vi "Tosca.vi"() -> ()   [LabVIEW 2020]
uses:
  Typedefs/Tosca-Control Refs.ctl
  FSM Graph VIs/LV Source/FSM Editor/FSM Editor.xctl
  Typedefs/Tosca-Thread Indicator.ctl
  FSM Graph VIs/LV Source/Classes/FSM.Graph/FSM.Graph.lvclass
  Typedefs/Tosca-State.ctl
  Typedefs/Tosca-Thread Type.ctl
  Typedefs/Tosca-General Options.ctl
  Classes/Parameters/Parameters.lvclass
  Classes/Parameters/Parameters.lvclass/Parameters.ctl
  Imaging VIs/Tosca-Imaging Mode.ctl
  Typedefs/Tosca-Schedule Mode.ctl
  Digital Input VIs/Tosca-DI Queue Data.ctl
  Digital Input VIs/Tosca-Input Event.ctl
  Digital Input VIs/Tosca-Input Criterion.ctl
  epl-vi-lib/Utility VIs/Type Defs/Logic State.ctl
  Typedefs/Tosca-Accumulator.ctl
  Classes/State/State.lvclass
  Classes/Parameters/Write Description.vi
  Classes/Parameters/Write MATLAB function.vi
  Classes/Parameters/Write Link to.vi
  Classes/Parameters/Read mode.vi
  8f5c66ef-750c-404f-9db0-703c45192de8.vi
  1561aa21-152f-4a32-afd8-a8b752fbf593.vi
  Classes/Parameters/Read Connect.vi
  Classes/Parameters/Write Connect.vi
  Classes/Parameters/Read AI.vi
  Classes/Parameters/Write AI.vi
  Classes/Parameters/Read Masker.vi
  Classes/Parameters/Read Use masker.vi
  Classes/Parameters/Write Masker.vi
  Classes/Parameters/Write Use masker.vi
  Classes/Parameters/Read Pretrial.vi
  Classes/Parameters/Read DAQ.vi
  Classes/Parameters/Write Pretrial.vi
  Classes/Parameters/Read Schedule Mode.vi
  Classes/Parameters/Read Imaging.vi
  Classes/Parameters/Write Imaging.vi
  Classes/Parameters/Read MATLAB function.vi
  Classes/Parameters/Read Input Events.vi
  Classes/Parameters/Read Flags.vi
  Classes/Parameters/Read Link to.vi
  Classes/Parameters/Write Flowchart.vi
  Sub VIs/Tosca-Globals.vi
  <vilib>/Utility/config.llb/Open Config Data.vi
  <vilib>/Utility/config.llb/Get Key Names.vi
  <vilib>/Utility/config.llb/Read Key.vi
  <vilib>/Utility/config.llb/Read Key (String).vi
  epl-vi-lib/Utility VIs/Array Manipulation VIs/String Array to Comma Separated String.vi
  <vilib>/Utility/error.llb/Error Cluster From Error Code.vi
  <vilib>/Utility/config.llb/Close Config Data.vi
  epl-vi-lib/Signal Synthesis VIs/4th Generation/Classes/SignalManager/SignalManager.lvclass
  epl-vi-lib/Signal Synthesis VIs/4th Generation/Classes/Channel/Channel.lvclass
  <vilib>/Platform/browser.llb/Open URL in Default Browser (path).vi
panel:
  out "play":bool
  in  "Link to":path
  out "FSM.Graph":refnum<class "FSM.Graph.lvclass">(xcontrol)
  in  "Pause":bool
  out "startAI":bool
  out "AI":errorcluster
  in  "Scripting":bool
  in  "Connect":bool
  in  "Sched:Seq":bool
  in  "Sched:2AFC":bool
  in  "Sched:CS+/CS-":bool
  in  "MATLAB function":path caption="MATLAB analysis function"
  out "2P":errorcluster
  out "FrameRate":dbl format="2P: %.5f Hz"
  out "Thread Indicators":T1[](array[typedef])
  out "DI dummy":picture
  in  "Cancel":bool
  in  "Apply":bool
  in  "Save as":bool
  in  "Analog Input":bool
  out "DI":errorcluster
  in  "Status":enum32{"CSStatus", "Adapt"}(tab)
  out "Slide":i32(slide) caption="Block 1/70:" scale=0.0..9.0
  out "Log":string
  in  "Graphs":enum32{"CSHist", "Adapt"}(tab)
  out "Histogram":cluster{dbl[], dbl[]}[](graph)
  out "Track":cluster{dbl[], dbl[]}[](graph) caption="Track1"
  out "finished":errorcluster
  in  "Imaging":bool
  out "SC":string
  in  "Masker":bool
  in  "Session Info":T2={"Subject ID"="", "Session"=1, "Path"=path "", "Run"=0} {"Session" min=1 step=1}
  in  "Notes":string
  in  "Result":string
  out "Control Refs":T3
  in  "General Options":bool
  in  "Play":bool
  in  "Flowchart":bool
  in  "Calibration":bool
  in  "Devices":bool
  in  "Save":bool
  in  "Open":bool
  in  "Exit":bool
  in  "Description":string
  in  "Parameter file":path
  out "Run":i32
  in  "Stop":bool
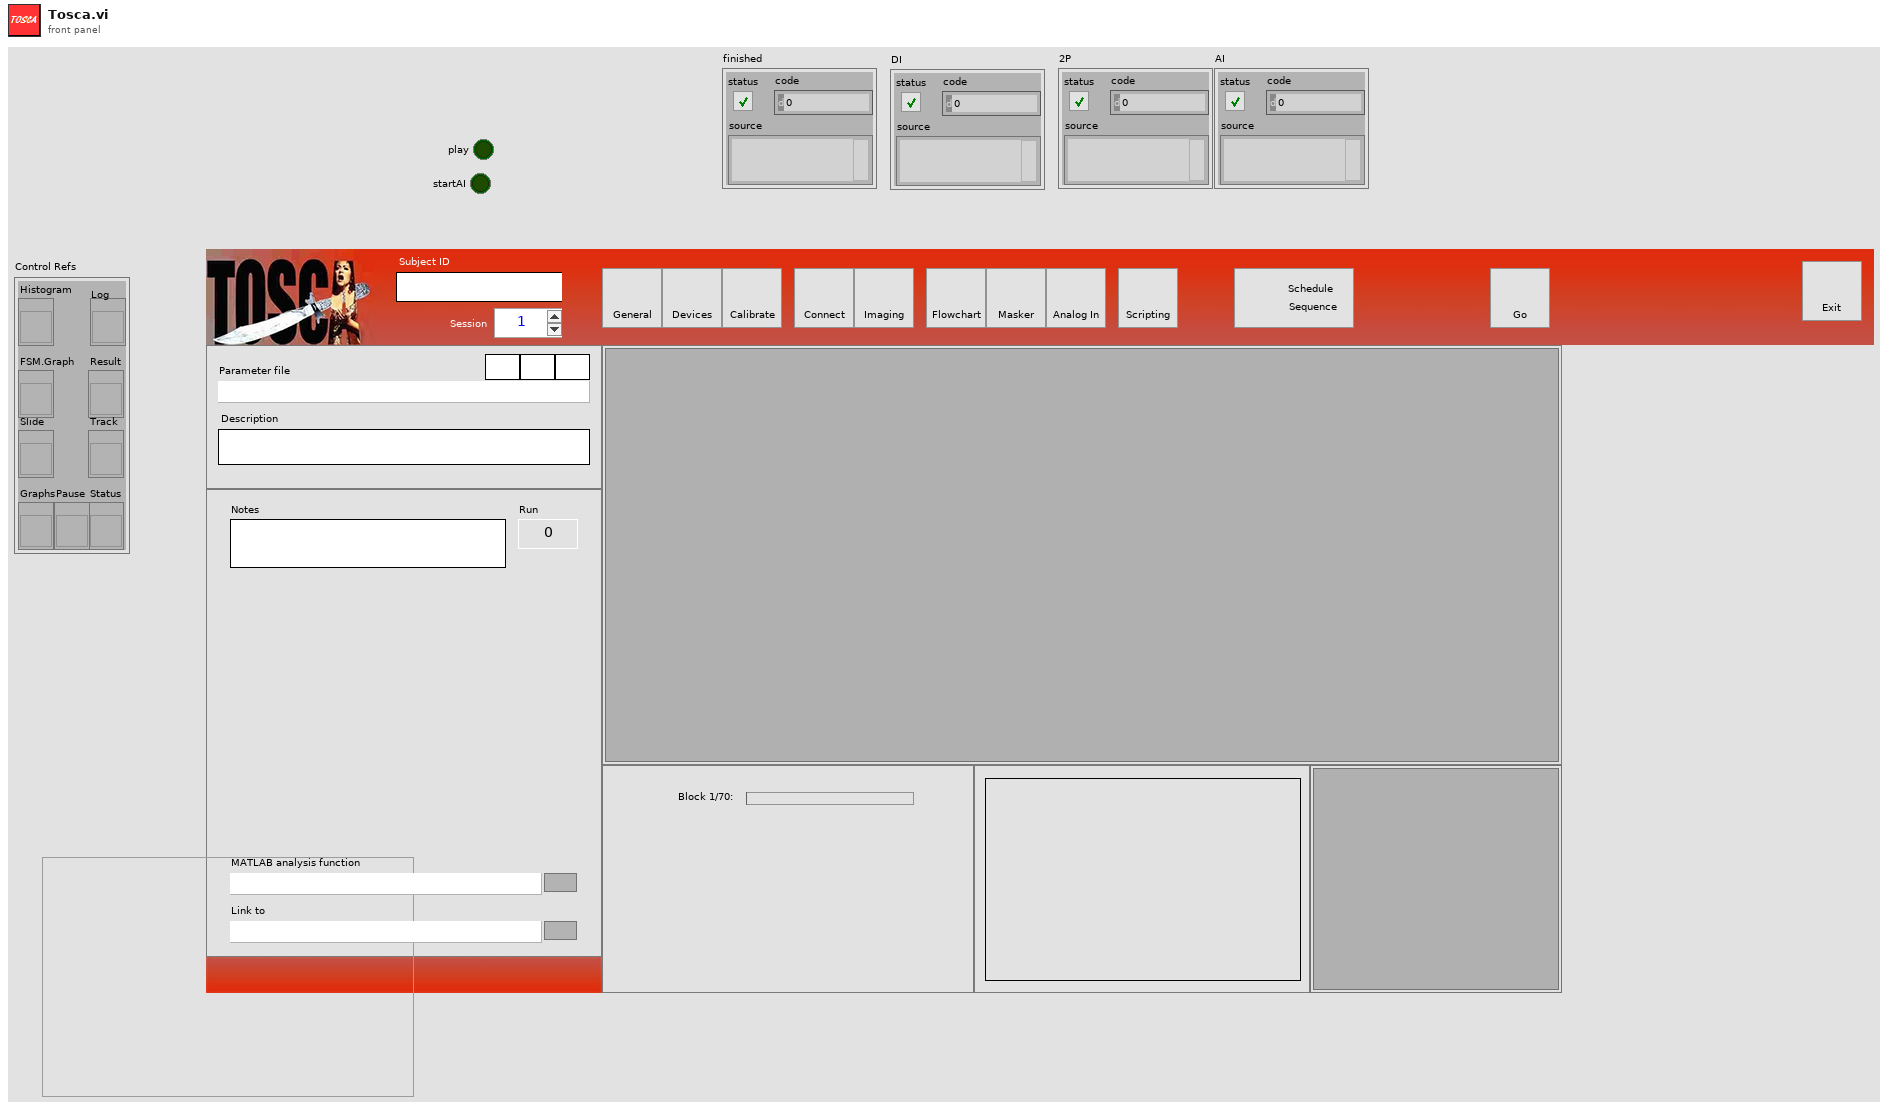
[diagram p1: front panel]
types:
  T1 = typedef "Tosca-Thread Indicator.ctl" = u16
  T2 = cluster{"Subject ID":string, "Session":i32, "Path":path, "Run":i32}
  T3 = typedef "Tosca-Control Refs.ctl" = cluster{"FSM.Graph":refnum<vi>, "Slide":refnum<vi>, "Result":refnum<vi>, "Histogram":refnum<vi>, "Graphs":refnum<vi>, "Track":refnum<vi>, "Log":refnum<vi>, "Status":refnum<vi>, "Pause":refnum<vi>}
  T4 = typedef "Tosca-State.ctl" = cluster{"Measuring":bool, "DI running":bool, "dirty":bool, "Restore":cluster{"Params":path}, "Session":cluster{"ID":string, "Num":i32, "Path":path, "Run":i32}, "active threads":T5[], "MATLAB":bool, "Config":path, "aborted":bool}
  T5 = typedef "Tosca-Thread Type.ctl" = enum16{"None", "AODO", "Masker", "ET", "Imaging", "Pupil", "AI", "DI", "Camera", "TTL out", "Loco", "Visual"}
  T6 = typedef "Tosca-IPC.ctl" = cluster{"Start":refnum<notifier>, "DI":refnum<queue>, "AO/DO":refnum<queue>, "Synapse":refnum<queue>, "Message":refnum<queue>, "Abort":refnum<notifier>, "Events":cluster{"DI":refnum<user-event>, "Threads ":refnum<user-event>}, "T/S/R":refnum<notifier>, "2P":refnum<notifier>, "MATLAB":refnum<notifier>, "Pupil":refnum<queue>, "Loco":refnum<queue>, "AI":refnum<queue>, "Tracking":refnum<queue>, "Visual":refnum<queue>, "File":refnum<notifier>}
  T7 = typedef "Tosca-2P-Notifier Data.ctl" = cluster{"Start":bool}
  T8 = typedef "Tosca-DI Queue Data.ctl" = cluster{"Action":enum16{"Stop", "Preview", "Run"}, "Input Events":T9[]}
  T9 = typedef "Tosca-Input Event.ctl" = cluster{"Name":string, "Criteria":T10[], "Operators":enum16{"AND", "OR"}[], "Accumulator":T12}
  T10 = typedef "Tosca-Input Criterion.ctl" = cluster{"DigInput":i32, "State":T11, "Time (ms)":i32, "Name":string}
  T11 = typedef "Logic State.ctl" = enum16{"Low", "High", "Rising", "Falling"}
  T12 = typedef "Tosca-Accumulator.ctl" = cluster{"active":bool, "N":i32, "T":dbl, "Imax":dbl, "latency":dbl}
  T13 = typedef "Tosca-State AODO.ctl" = cluster{"Name":string, "T (s)":dbl, "First AO":dbl[][], "frames/rep":i32, "finish?":bool, "Nrep":i32, "AO":T14, "DO":T15, "immediate":bool, "First DO":bool[][], "SigMan":refnum<class "SignalManager.lvclass">}
  T14 = typedef "Tosca-AO Runtime.ctl" = cluster{"Fs (Hz)":dbl, "pts/frame":i32, "pts/rep":i32, "ramp off":bool[], "fade out":dbl[][]}
  T15 = typedef "Tosca-DO Runtime.ctl" = cluster{"Fs (Hz)":dbl, "pts/frame":i32, "pts/rep":i32, "Rep":i32, "State":i32, "Trial":i32, "Frame":i32, "frOut":bool[], "Nchan":i32}
  T16 = typedef "Tosca-Synapse Start Data.ctl" = cluster{"Path":path, "Codes":string, "retrieve":bool}
  T17 = typedef "Tosca-SG Runtime Params.ctl" = cluster{"AO":T14, "DO":T15, "image":T18}
  T18 = typedef "Tosca-Imaging Mode.ctl" = enum16{"Off", "Widefield", "Two-photon"}
  T19 = typedef "Tosca-Session Info.ctl" = cluster{"Animal ID":string, "Session":i32, "Path":path, "Run":i32}
  T20 = typedef "Tosca-Analysis State.ctl" = cluster{"Path":path, "Attempted":i32, "Adapt":T21, "MATLAB function":path, "Results":T24[], "group order":i32[], "Connect":T25}
  T21 = typedef "Tosca-Adaptation State.ctl" = cluster{"which":i32, "nacq":i32, "Tracks":T22[]}
  T22 = typedef "Tosca-Adaptation Track State.ctl" = cluster{"Value":dbl, "Ncorrect":i32, "Nrev":i32, "Prev":dbl, "History":T23[], "Threshold":dbl, "last":i32, "type":string, "catches":dbl[][], "name":string}
  T23 = typedef "Tosca-Adaptation History Element.ctl" = cluster{"Value":dbl, "Result":string, "Log":string, "reversal":bool, "Catch":dbl}
  T24 = typedef "Parameters.lvclass/Histogram Data.ctl" = cluster{"Family":string, "Names":string[], "Colors":u32[], "N":i32[]}
  T25 = typedef "Parameters.lvclass/Connect.ctl" = cluster{"Tracking":bool, "Synapse":bool, "Pupil":bool, "Loco":bool, "Retrieve":bool, "Codes":string}
  T26 = typedef "Tosca-SCL Element.ctl" = cluster{"name":string, "vars":cluster{"state":string, "chan":string, "param":string, "value":dbl}[], "text":string, "mode":T27, "family":string, "type":T28}
  T27 = typedef "Tosca-Schedule Mode.ctl" = enum16{"Seq", "CS+/CS-", "Adapt"}
  T28 = typedef "Tosca-Event Type.ctl" = enum16{"Normal", "CS+", "CS-"}
  T29 = typedef "Tosca-Trial Result Enum.ctl" = enum16{"No trial", "Go", "No go", "Error", "Abort"}
  T30 = enum16{"big-endian, network order", "native, host order", "little-endian"}
  T31 = enum8{"Enabled", "Disabled", "Disabled and Grayed Out"}
  T32 = typedef "Tosca-General Options.ctl" = cluster{"AutoDI":bool, "Max errors":i32, "Headway (%)":dbl, "DI dt":i32}
  T33 = typedef "Tosca-Visual Display Settings.ctl" = cluster{"Use PTB":bool, "IP Address":string, "Port":i32, "rect":cluster{"left":i16, "top":i16, "width":i16, "height":i16}, "Full screen":bool, "Open at start":bool, "Monitor":i32, "Monitor size (in)":dbl, "Monitor dist (in)":dbl, "Photodiode Square":cluster{"size":i16, "location":enum16{"Bottom Left", "Top Left", "Top Right", "Bottom Right"}}, "Background":dbl}
  T34 = cluster{"FSM.Graph":refnum<vi>, "Slide":refnum<vi>, "Result":refnum<vi>, "Histogram":refnum<vi>, "Graphs":refnum<vi>, "Track":refnum<vi>, "Log":refnum<vi>, "Status":refnum<vi>, "Pause":refnum<vi>}
  T35 = cluster{"ID":string, "Num":i32, "Path":path, "Run":i32}
  T36 = typedef "Tosca-AI.ctl" = cluster{"active":bool, "Fs":dbl, "AI":string[], "DI":string[]}
  T37 = typedef "Tosca-Pretrial Spec.ctl" = cluster{"Path":path, "Args":string[]}
  T38 = typedef "Parameters.lvclass/DAQ.ctl" = cluster{"AO Fs (Hz)":dbl, "DO Fs (Hz)":dbl, "Poll Rate (Hz)":dbl, "Baseline (s)":dbl}
  T39 = typedef "Tosca-Imaging.ctl" = cluster{"mode":T18, "FrameRateHz":dbl, "use AO":bool, "destination":string}
  T40 = typedef "Tosca-Flag.ctl" = cluster{"Name":string, "Default":i32}
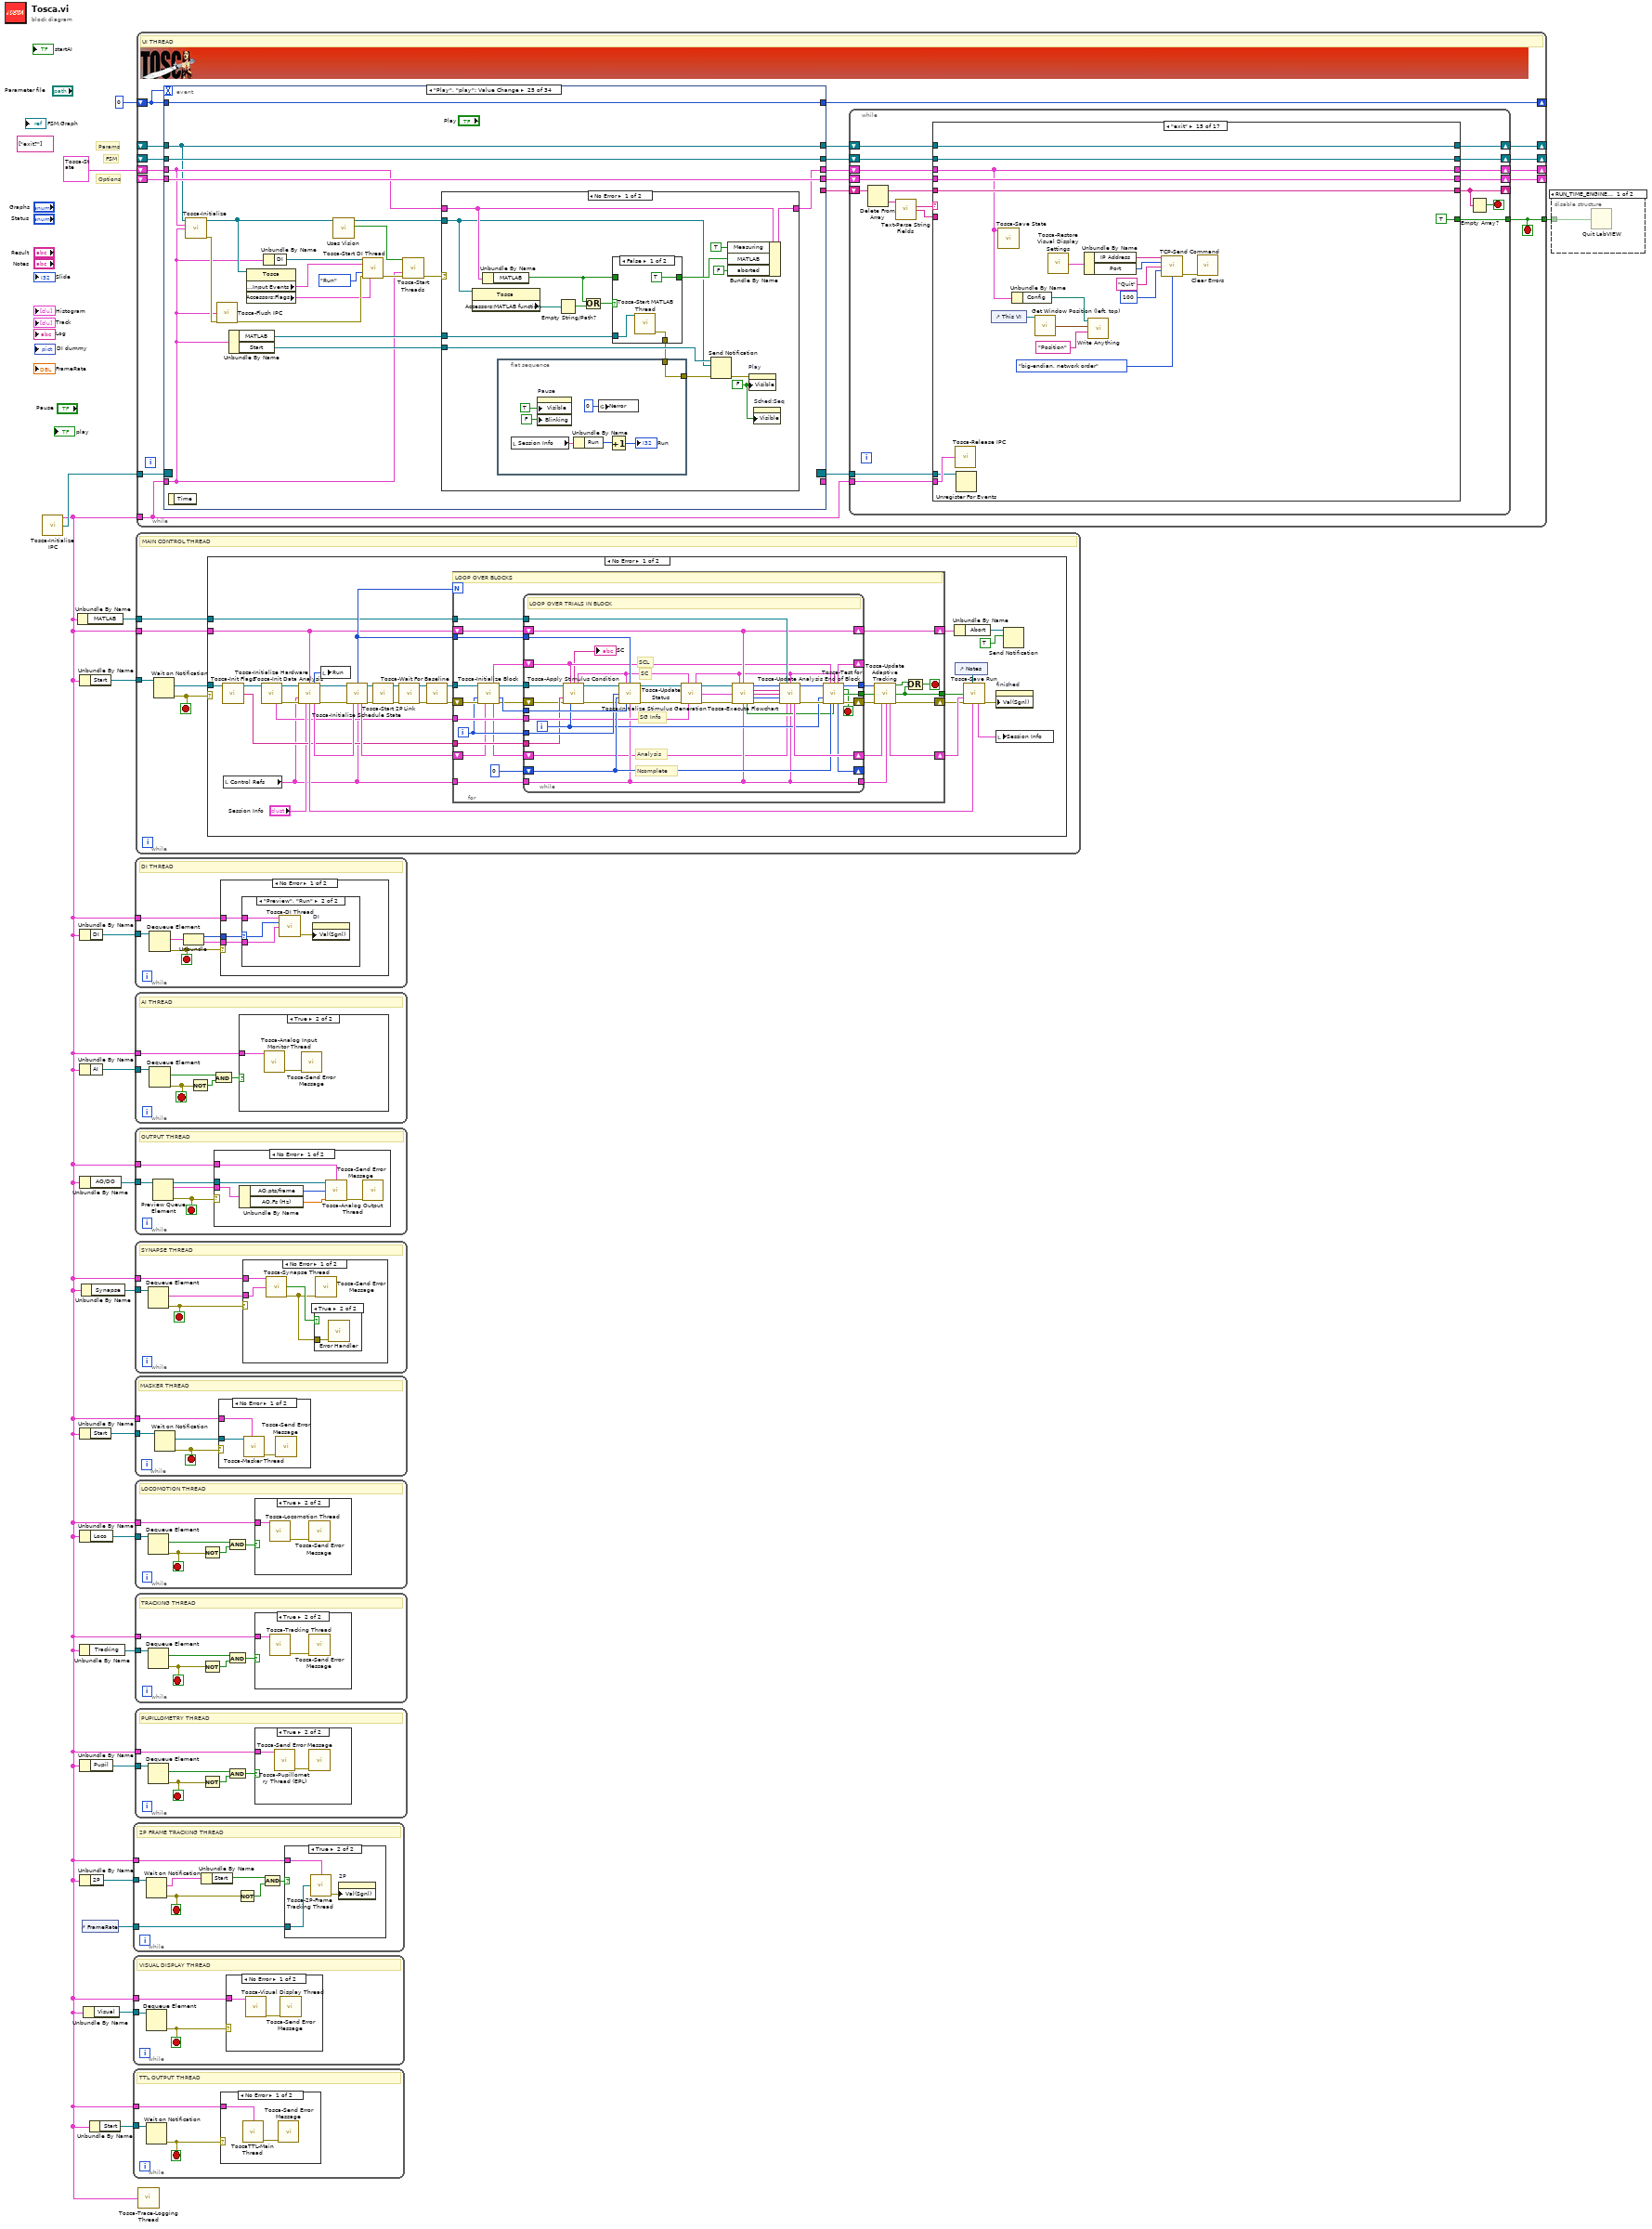
[diagram p0: block diagram]
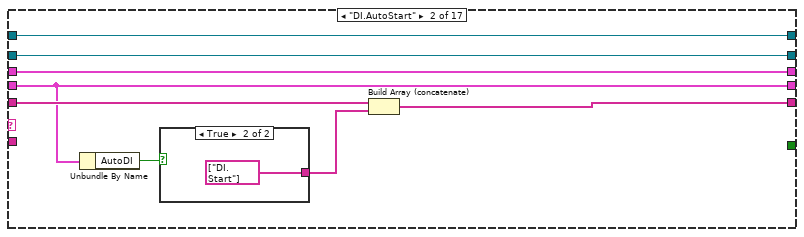
[diagram p5: hidden frame]
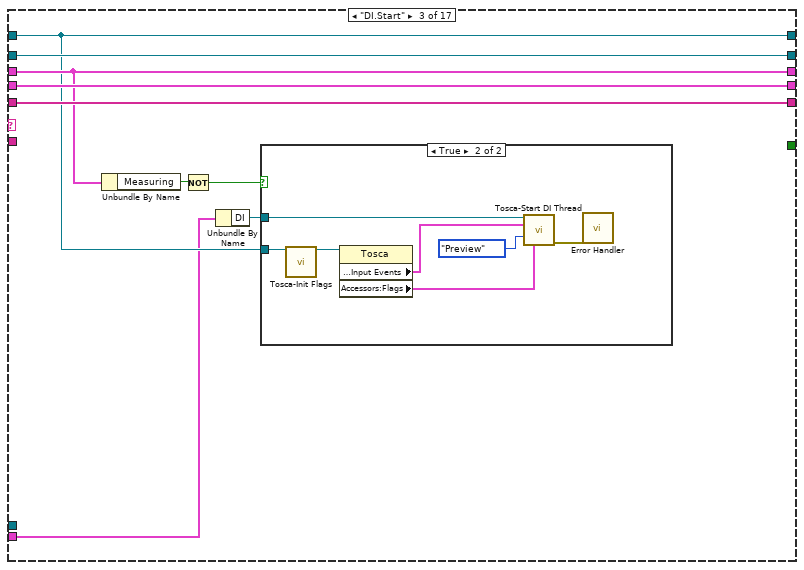
[diagram p7: hidden frame]
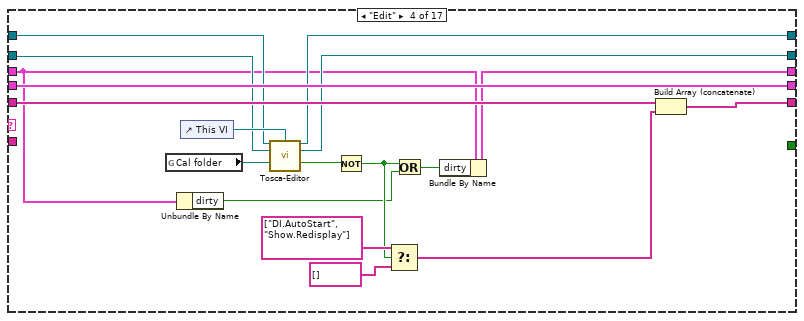
[diagram p9: hidden frame]
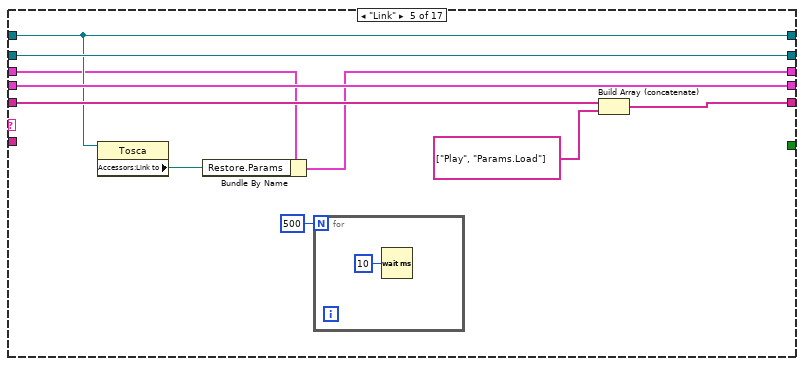
[diagram p10: hidden frame]
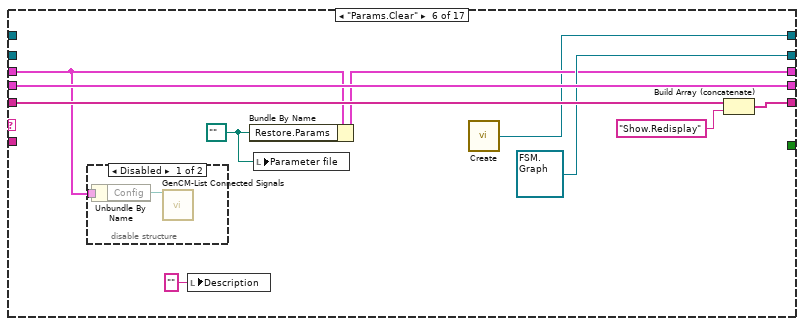
[diagram p11: hidden frame]
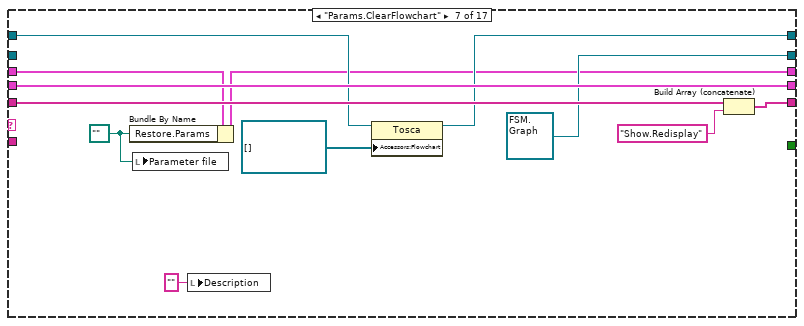
[diagram p13: hidden frame]
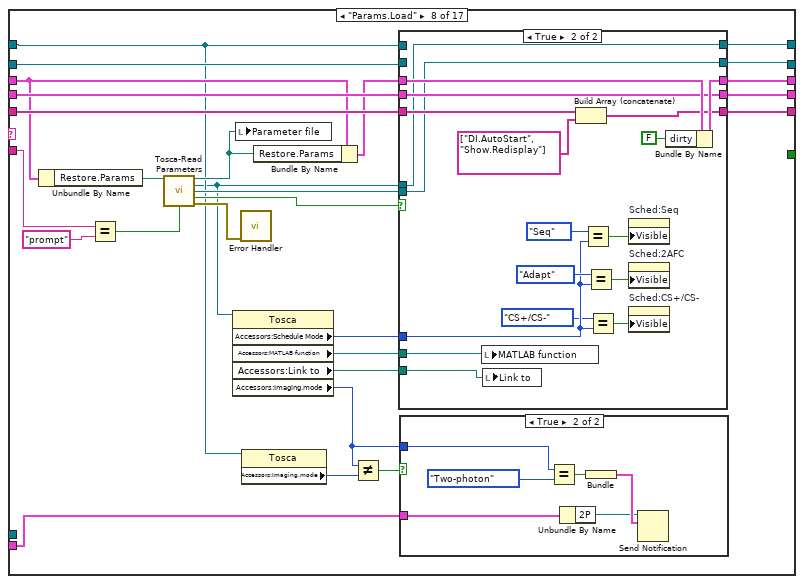
[diagram p14: hidden frame]
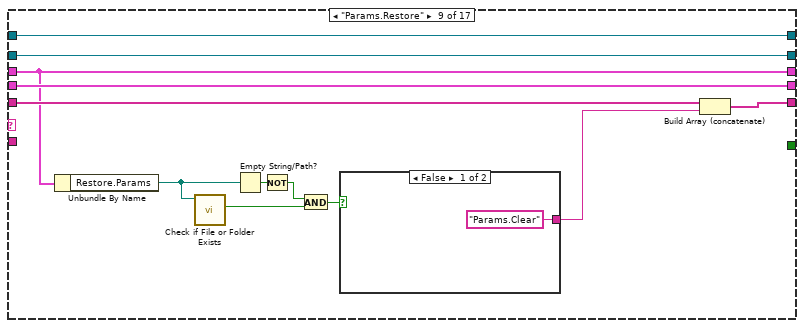
[diagram p17: hidden frame]
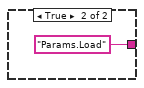
[diagram p18: hidden frame]
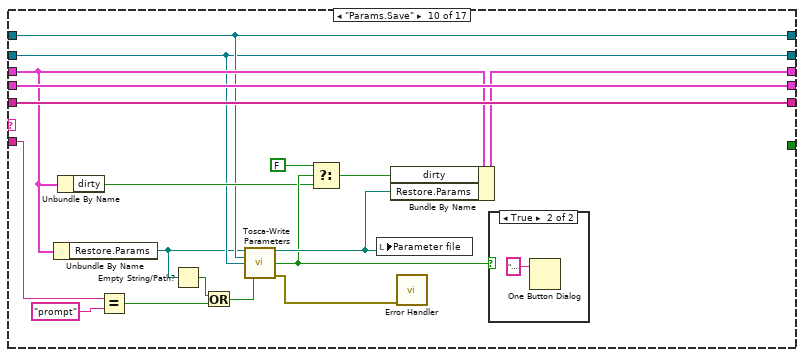
[diagram p19: hidden frame]
diagram:
  (unwired) string[] ["exit?"]
  # "FSM"
  # "Params"
  # "Options"
  n1 = call "Tosca-Initialize IPC.vi"() -> ("IPC"=w1:T6, "Event Registration Refnum"=w11:refnum<event-registration>)  [unwired: 13 in, 1 out]
  n2 = Unbundle By Name(w1) -> ("MATLAB"=w8:refnum<notifier>)
  n3 = Unbundle By Name(w1) -> ("Tracking"=w3:refnum<queue>)
  n4 = Unbundle By Name(w1) -> ("Start"=w17:refnum<notifier>)
  n5 = Unbundle By Name(w1) -> ("DI"=w14:refnum<queue>)
  n6 = Unbundle By Name(w1) -> ("AI"=w4:refnum<queue>)
  n7 = Unbundle By Name(w1) -> ("AO/DO"=w13:refnum<queue>)
  n8 = Unbundle By Name(w1) -> ("Start"=w15:refnum<notifier>)
  n9 = Unbundle By Name(w1) -> ("Loco"=w5:refnum<queue>)
  n10 = Unbundle By Name(w1) -> ("Pupil"=w6:refnum<queue>)
  n11 = Unbundle By Name(w1) -> ("2P"=w10:refnum<notifier>)
  n12 = Unbundle By Name(w1) -> ("Synapse"=w16:refnum<queue>)
  n13 = control-ref of="FrameRate"() -> (w9:refnum<vi>)
  n14 = Unbundle By Name(w1) -> ("Visual"=w2:refnum<queue>)
  n15 = Unbundle By Name(w1) -> ("Start"=w7:refnum<notifier>)
  n16 = while {
    tunnel: w10 -> [w27]
    tunnel: w1 -> [w21]
    tunnel: w9 -> [w20]
    stop <- w22 stop-if-true
    # "2P FRAME TRACKING THREAD"
    n17 = Wait on Notification(notifier=w27) -> (notification=w26:T7, error out=w22:errorcluster)  [unwired: 3 in, 2 out]
    n18 = Unbundle By Name(w26) -> ("Start"=w24:bool)
    n19 = Not(x=w22) -> (.not. x?=w23:bool)
    n20 = And(x=w24, y=w23) -> (x .and. y?=w25:bool)
    n21 = case shown="True" w25 {
      tunnel: w21 -> [_ w30]
      tunnel: w20 -> [_ w29]
      frame False {
      }
      frame True {
        n22 = call "Tosca-2P-Frame Tracking Thread.vi"("IPC"=w30, "FrameRate"=w29) -> ("error out"=w28:errorcluster)  [unwired: 13 in]
        n23 = property on="2P" class="Clust (strict)"("Val(Sgnl)"=w28) -> ()  [unwired: 2 in, 2 out]
      }
    }
  }
  n24 = while {
    tunnel: w2 -> [w33]
    tunnel: w1 -> [w32]
    stop <- w31 stop-if-true
    # "VISUAL DISPLAY THREAD"
    n25 = Dequeue Element(queue=w33) -> (error out=w31:errorcluster)  [unwired: 2 in, 3 out]
    n26 = case shown="No Error" w31 {
      tunnel: w32 -> [w34 _]
      frame No Error {
        n27 = call "Tosca-Visual Display Thread.vi"("IPC"=w34) -> ("error out"=w35:errorcluster)  [unwired: 14 in]
        n28 = call "Tosca-Send Error Message.vi"("error in (no error)"=w35) -> ()  [unwired: 15 in]
      }
      frame Error {
      }
    }
  }
  n29 = while {
    tunnel: w7 -> [w38]
    tunnel: w1 -> [w37]
    stop <- w36 stop-if-true
    # "TTL OUTPUT THREAD"
    n30 = Wait on Notification(notifier=w38) -> (error out=w36:errorcluster)  [unwired: 3 in, 3 out]
    n31 = case shown="No Error" w36 {
      tunnel: w37 -> [w40 _]
      frame No Error {
        n32 = call "ToscaTTL-Main Thread.vi"("IPC"=w40) -> ("error out"=w39:errorcluster)  [unwired: 14 in]
        n33 = call "Tosca-Send Error Message.vi"("error in (no error)"=w39) -> ()  [unwired: 15 in]
      }
      frame Error {
      }
    }
  }
  n34 = while {
    tunnel: w15 -> [w44]
    tunnel: w1 -> [w41]
    stop <- w43 stop-if-true
    # "MASKER THREAD"
    n35 = Wait on Notification(notifier=w44) -> (notification=w42:refnum<class "Parameters.lvclass">, error out=w43:errorcluster)  [unwired: 3 in, 2 out]
    n36 = case shown="No Error" w43 {
      tunnel: w42 -> [w47 _]
      tunnel: w41 -> [w45 _]
      frame No Error {
        n37 = call "Tosca-Masker Thread.vi"("IPC"=w45, "Tosca"=w47) -> ("error out"=w46:errorcluster)  [unwired: 9 in]
        n38 = call "Tosca-Send Error Message.vi"("error in (no error)"=w46) -> ()  [unwired: 15 in]
      }
      frame Error {
      }
    }
  }
  n39 = while {
    tunnel: w14 -> [w52]
    tunnel: w1 -> [w53]
    stop <- w49 stop-if-true
    # "DI THREAD"
    n40 = Dequeue Element(queue=w52) -> (element=w51:T8, error out=w49:errorcluster)  [unwired: 2 in, 2 out]
    n41 = Unbundle(w51) -> ("Action"=w48:enum16{"Stop", "Preview", "Run"}, "Input Events"=w50:T9[])
    n42 = case shown="No Error" w49 {
      tunnel: w53 -> [w56 _]
      tunnel: w50 -> [w55 _]
      tunnel: w48 -> [w54 _]
      frame No Error {
        n43 = case shown="\"Preview\", \"Run\"" w54 {
          selector: w54 -> [_ w57]
          tunnel: w56 -> [_ w60]
          tunnel: w55 -> [_ w59]
          frame "Stop", Default {
          }
          frame "Preview", "Run" {
            n44 = call "Tosca-DI Thread.vi"("IPC"=w60, "Action"=w57, "Input Events"=w59) -> ("error out"=w58:errorcluster)  [unwired: 12 in]
            n45 = property on="DI" class="Clust (strict)"("Val(Sgnl)"=w58) -> ()  [unwired: 2 in, 2 out]
          }
        }
      }
      frame Error {
      }
    }
  }
  n46 = while {
    tunnel: w4 -> [w65]
    tunnel: w1 -> [w66]
    stop <- w62 stop-if-true
    # "AI THREAD"
    n47 = Dequeue Element(queue=w65) -> (element=w63:bool, error out=w62:errorcluster)  [unwired: 2 in, 2 out]
    n48 = Not(x=w62) -> (.not. x?=w61:bool)
    n49 = And(x=w63, y=w61) -> (x .and. y?=w64:bool)
    n50 = case shown="True" w64 {
      tunnel: w66 -> [_ w68]
      frame False {
      }
      frame True {
        n51 = call "Tosca-Analog Input Monitor Thread.vi"("IPC"=w68) -> ("error out"=w67:errorcluster)  [unwired: 14 in]
        n52 = call "Tosca-Send Error Message.vi"("error in (no error)"=w67) -> ()  [unwired: 15 in]
      }
    }
  }
  n53 = while {
    tunnel: w13 -> [w73]
    tunnel: w1 -> [w71]
    stop <- w69 stop-if-true
    # "OUTPUT THREAD"
    n54 = Preview Queue Element(queue=w73) -> (queue out=w72:refnum<queue>, element=w70:T13, error out=w69:errorcluster)  [unwired: 2 in, 1 out]
    n55 = case shown="No Error" w69 {
      tunnel: w72 -> [w79 _]
      tunnel: w71 -> [w78 _]
      tunnel: w70 -> [w76 _]
      frame No Error {
        n56 = Unbundle By Name(w76) -> ("AO.pts/frame"=w75:i32, "AO.Fs (Hz)"=w74:dbl)
        n57 = call "Tosca-Analog Output Thread.vi"("Tosca Output Queue"=w79, "IPC"=w78, "pts/frame"=w75, "Fs (Hz)"=w74) -> ("error out"=w77:errorcluster)  [unwired: 11 in]
        n58 = call "Tosca-Send Error Message.vi"("error in (no error)"=w77) -> ()  [unwired: 15 in]
      }
      frame Error {
      }
    }
  }
  n59 = while {
    tunnel: w16 -> [w83]
    tunnel: w1 -> [w81]
    stop <- w82 stop-if-true
    # "SYNAPSE THREAD"
    n60 = Dequeue Element(queue=w83) -> (element=w80:T16, error out=w82:errorcluster)  [unwired: 2 in, 2 out]
    n61 = case shown="No Error" w82 {
      tunnel: w81 -> [w87 _]
      tunnel: w80 -> [w84 _]
      frame No Error {
        n62 = call "Tosca-Synapse Thread.vi"("IPC"=w87, "Data"=w84) -> ("aborted"=w86:bool, "error out"=w85:errorcluster)  [unwired: 12 in]
        n63 = case shown="True" w86 {
          tunnel: w85 -> [_ w88]
          frame False {
          }
          frame True {
            n64 = call "Error Handler.vi"("error in (no error)"=w88) -> ()  [unwired: 12 in, 3 out]
          }
        }
        n65 = call "Tosca-Send Error Message.vi"("error in (no error)"=w85) -> ()  [unwired: 15 in]
      }
      frame Error {
      }
    }
  }
  n66 = while {
    tunnel: w5 -> [w94]
    tunnel: w1 -> [w93]
    stop <- w91 stop-if-true
    # "LOCOMOTION THREAD"
    n67 = Dequeue Element(queue=w94) -> (element=w90:bool, error out=w91:errorcluster)  [unwired: 2 in, 2 out]
    n68 = Not(x=w91) -> (.not. x?=w92:bool)
    n69 = And(x=w90, y=w92) -> (x .and. y?=w89:bool)
    n70 = case shown="True" w89 {
      tunnel: w93 -> [_ w96]
      frame False {
      }
      frame True {
        n71 = call "Tosca-Locomotion Thread.vi"("IPC"=w96) -> ("error out"=w95:errorcluster)  [unwired: 14 in]
        n72 = call "Tosca-Send Error Message.vi"("error in (no error)"=w95) -> ()  [unwired: 15 in]
      }
    }
  }
  n73 = while {
    tunnel: w3 -> [w97]
    tunnel: w1 -> [w102]
    stop <- w100 stop-if-true
    # "TRACKING THREAD"
    n74 = Dequeue Element(queue=w97) -> (element=w99:bool, error out=w100:errorcluster)  [unwired: 2 in, 2 out]
    n75 = Not(x=w100) -> (.not. x?=w101:bool)
    n76 = And(x=w99, y=w101) -> (x .and. y?=w98:bool)
    n77 = case shown="True" w98 {
      tunnel: w102 -> [_ w104]
      frame False {
      }
      frame True {
        n78 = call "Tosca-Tracking Thread.vi"("IPC"=w104) -> ("error out"=w103:errorcluster)  [unwired: 14 in]
        n79 = call "Tosca-Send Error Message.vi"("error in (no error)"=w103) -> ()  [unwired: 15 in]
      }
    }
  }
  n80 = while {
    tunnel: w6 -> [w110]
    tunnel: w1 -> [w109]
    stop <- w107 stop-if-true
    # "PUPILLOMETRY THREAD"
    n81 = Dequeue Element(queue=w110) -> (element=w106:bool, error out=w107:errorcluster)  [unwired: 2 in, 2 out]
    n82 = Not(x=w107) -> (.not. x?=w108:bool)
    n83 = And(x=w106, y=w108) -> (x .and. y?=w105:bool)
    n84 = case shown="True" w105 {
      tunnel: w109 -> [_ w111]
      frame False {
      }
      frame True {
        n85 = call "Tosca-Pupillometry Thread (EPL).vi"("IPC"=w111) -> ("error out"=w112:errorcluster)  [unwired: 14 in]
        n86 = call "Tosca-Send Error Message.vi"("error in (no error)"=w112) -> ()  [unwired: 15 in]
      }
    }
  }
  n87 = while {
    tunnel: w17 -> [w117]
    tunnel: w1 -> [w114]
    tunnel: w8 -> [w113]
    stop <- w115 stop-if-true
    # "MAIN CONTROL THREAD"
    n88 = Wait on Notification(notifier=w117) -> (notification=w116:refnum<class "Parameters.lvclass">, error out=w115:errorcluster)  [unwired: 3 in, 2 out]
    n89 = case shown="No Error" w115 {
      tunnel: w116 -> [w133 _]
      tunnel: w114 -> [w119 _]
      tunnel: w113 -> [w137 _]
      frame No Error {
        n90 = call "Tosca-Init Flags.vi"("Tosca"=w133) -> ("Tosca Out"=w132:refnum<class "Parameters.lvclass">, "Names"=w135:string[])  [unwired: 13 in]
        n91 = local read "Control Refs"() -> (w118:T3)
        n92 = call "Tosca-Initialize Hardware.vi"("Tosca"=w132) -> ("Tosca out"=w130:refnum<class "Parameters.lvclass">, "SG Runtime"=w131:T17, "error out"=w124:errorcluster)  [unwired: 12 in]
        n93 = call "Tosca-Init Data Analysis.vi"("Tosca"=w130, "IPC"=w119, "Control Refs"=w118, "error in (no error)"=w124, "Session Info"="Session Info") -> ("Run"=w125:i32, "Tosca out"=w129:refnum<class "Parameters.lvclass">, "Session Info out"=w147:T19, "Analysis"=w142:T20, "error out"=w144:errorcluster)  [unwired: 6 in]
        n94 = local write "Run"(w125) -> ()
        n95 = call "Tosca-Initialize Schedule State.vi"("Tosca"=w129, "error in (no error)"=w144, "Analysis In"=w142, "Controls"=w118) -> ("Blocks"=w145:i32, "Tosca out"=w128:refnum<class "Parameters.lvclass">, "Analysis Out"=w141:T20, "error out"=w143:errorcluster)  [unwired: 8 in]
        n96 = call "Tosca-Start 2P.vi"("Tosca"=w128, "error in (no error)"=w143) -> ("Tosca out"=w127:refnum<class "Parameters.lvclass">, "error out"=w126:errorcluster)  [unwired: 12 in]
        n97 = call "Link.vi"("Tosca in"=w127, "error in (no error)"=w126) -> ("Tosca out"=w122:refnum<class "Parameters.lvclass">, "error out"=w120:errorcluster)  [unwired: 12 in]
        n98 = call "Tosca-Wait For Baseline.vi"("Parameters in"=w122, "error in (no error)"=w120) -> ("Parameters out"=w123:refnum<class "Parameters.lvclass">, "error out"=w121:errorcluster)  [unwired: 12 in]
        n99 = for {
          N: w145 -> [_]
          tunnel: w131 -> [w177]
          tunnel: w118 -> [w176]
          tunnel: w145 -> [w175]
          shift-right: [w171] -> w150
          shift-left: w141 -> [w157]
          tunnel: [w167] -> w148
          shift-right: [w169] -> w146
          shift-left: w121 -> [w178]
          shift-right: [w163] -> w140
          shift-left: w119 -> [w162]
          tunnel: w137 -> [w161]
          tunnel: w135 -> [w160]
          tunnel: w123 -> [w154]
          i -> [w159]
          stop <- w166 stop-if-true
          # "LOOP OVER BLOCKS"
          n100 = call "Tosca-Initialize Block.vi"("Tosca"=w154, "block"=w159, "error in (no error)"=w178, "Analysis in"=w157) -> ("SCL"=w152:T26[], "Tosca out"=w153:refnum<class "Parameters.lvclass">, "NumTrials"=w158:i32, "Analysis out"=w156:T20, "error out"=w155:errorcluster)  [unwired: 7 in]
          n101 = while {
            tunnel: w177 -> [w196]
            tunnel: w176 -> [w191]
            tunnel: w159 -> [w207]
            tunnel: w175 -> [w215]
            tunnel: w158 -> [w214]
            shift-right: [w211] -> w172
            shift-left: w156 -> [w190]
            tunnel: [w209] -> w170
            shift-right: [w208] -> _
            shift-left: w152 -> [w188]
            shift-right: [w204] -> _
            shift-left: 0 -> [w203]
            shift-right: [w212] -> w173
            shift-left: w155 -> [w194]
            tunnel: [w201] -> w165
            tunnel: [w191] -> w164
            shift-right: [w193] -> w163
            shift-left: w162 -> [w193]
            tunnel: w161 -> [w199]
            tunnel: w160 -> [w195]
            tunnel: w153 -> [w189]
            i -> [w200]
            stop <- w205 stop-if-true
            # "SG Info"
            # "Analysis"
            # "Ncomplete"
            # "SC"
            # "SCL"
            # "LOOP OVER TRIALS IN BLOCK"
            n102 = call "Tosca-Apply Stimulus Condition.vi"("Tosca"=w189, "SCL"=w188, "Flag names"=w195, "error in (no error)"=w194, "SCL index"=w200) -> ("text"=→"SC":string, "StimCon Element"=w180:T26, "Tosca out"=w186:refnum<class "Parameters.lvclass">, "error out"=w192:errorcluster)  [unwired: 7 in]
            n103 = call "Tosca-Update Status.vi"("StimCon"=w180, "NumBlocks"=w215, "Current Block"=w207, "This trial"=w203, "error in (no error)"=w192, "NumTrials"=w214, "Control Refs"=w191) -> ("error out"=w216:errorcluster)  [unwired: 8 in]
            n104 = call "Tosca-Initialize Stimulus Generation.vi"("Tosca"=w186, "StimCon in"=w180, "error in (no error)"=w216, "SG Runtime"=w196) -> ("StimCon out"=w179:T26, "Tosca out"=w185:refnum<class "Parameters.lvclass">, "AODO"=w184:T13[], "error out"=w181:errorcluster)  [unwired: 8 in]
            n105 = call "Tosca-Execute Flowchart.vi"("Tosca"=w185, "StimCon"=w179, "IPC"=w193, "AODO"=w184, "error in"=w181, "Control Refs"=w191) -> ("Result"=w210:T29, "History"=w202:string[], "Result string"=w198:string, "Rxn time"=w183:i32, "Abort"=w197:bool, "error out"=w182:errorcluster)  [unwired: 4 in]
            n106 = call "Tosca-Update Analysis.vi"("Result"=w210, "MATLAB"=w199, "StimCon Element"=w179, "History"=w202, "Result String"=w198, "Rxn time"=w183, "error in (no error)"=w182, "Analysis"=w190, "Control Refs"=w191) -> ("Result thru"=w206:T29, "Analysis out"=w211:T20, "error out"=w213:errorcluster)  [unwired: 4 in]
            n107 = call "Tosca-Test for End of Block.vi"("Result"=w206, "SCL in"=w188, "StimCon Element"=w179, "sclIndex"=w200, "error in (no error)"=w213, "Ncomplete"=w203, "Abort"=w197) -> ("SCL out"=w208:T26[], "Result thru"=w201:T29, "End block?"=w205:bool, "Abort?"=w209:bool, "Ncomplete out"=w204:i32, "error out"=w212:errorcluster)  [unwired: 3 in]
          }
          n108 = call "Tosca-Update Adaptive Tracking.vi"("Result"=w165, "Abort? in"=w170, "error in (no error)"=w173, "Analysis In"=w172, "Controls"=w164) -> ("Finished"=w168:bool, "Abort? out"=w167:bool, "Analysis Out"=w171:T20, "error out"=w169:errorcluster)  [unwired: 7 in]
          n109 = Or(x=w168, y=w167) -> (x .or. y?=w166:bool)
        }
        n110 = Unbundle By Name(w140) -> ("Abort"=w139:refnum<notifier>)
        n111 = control-ref of="Notes"() -> (w136:refnum<vi>)
        n112 = call "Tosca-Save Run.vi"("Notes"=w136, "Abort?"=w148, "Analysis"=w150, "error in (no error)"=w146, "Session Info"=w147) -> ("Session Info out"=w149:T19, "error out"=w151:errorcluster)  [unwired: 8 in, 1 out]
        n113 = property on="finished" class="Clust (strict)"("Val(Sgnl)"=w151) -> ()  [unwired: 2 in, 2 out]
        n114 = local write "Session Info"(w149) -> ()
        n115 = Send Notification(notification=TRUE, notifier=w139) -> ()  [unwired: 1 in, 2 out]
      }
      frame Error {
      }
    }
  }
  n116 = while {
    shift-right: [w235] -> _
    shift-left: 0 -> [w233]
    shift-right: [w220] -> _
    shift-left: _ -> [w222]
    shift-right: [w227] -> _
    shift-left: T4 {"Measuring"=FALSE, "DI running"=FALSE, "dirty"=FALSE, "Restore"={"Params"=path ""}, "Session"={"ID"="", "Num"=0, "Path"=path "", "Run"=0}, "active threads"=[], "MATLAB"=FALSE, "Config"=path "", "aborted"=FALSE} ("State") -> [w234]
    tunnel: [w225] -> w18
    tunnel: w1 -> [w223]
    shift-right: [w226] -> _
    shift-left: _ -> [w232]
    tunnel: w11 -> [w231]
    shift-right: [w218] -> _
    shift-left: _ -> [w217]
    stop <- w225 stop-if-true
    # "UI THREAD"
    n117 = event shown="[24] \"Play\", \"play\": Value Change" {
      selector: w231 -> [_ _ _ _ _ _ _ _ _ _ _ _ _ _ _ _ _ _ _ _ _ _ _ _ _ _ _ _ _ _ _ _ _ _]
      dyn-events: [_ _ _ _ _ _ _ _ _ _ _ _ _ _ _ _ _ _ _ _ _ _ _ _ _ _ _ _ _ _ _ _ _ _] -> w224
      timeout: w233 -> [_ _ _ _ _ _ _ _ _ _ _ _ _ _ _ _ _ _ _ _ _ _ _ _ _ _ _ _ _ _ _ _ _ _]
      tunnel: [-1 w602 w613 w617 w683 w687 w697 w703 w709 w715 w720 w729 w738 w747 w762 w800 w828 w859 w865 w879 w899 w918 w935 w956 w980 w1015 w1044 w1089 w1096 w1107 w1122 w1133 w1170 w1202] -> w235
      tunnel: w222 -> [_ w607 w614 w615 w682 w690 w696 w702 w708 w714 w718 w727 w736 w751 w766 w794 w830 w847 w864 w870 w894 w909 w922 w942 w966 w1018 w1031 w1088 w1095 w1106 w1121 w1132 w1152 w1201]
      tunnel: [refnum<class "Parameters.lvclass"> refnum ("Tosca") w607 w614 w615 w682 w690 w696 w702 w708 w714 w716 w725 w735 w751 w757 w795 w830 w848 w864 w866 w890 w903 w920 w936 w966 w1018 w1031 w1088 w1095 w1106 w1121 w1132 w1152 w1201] -> w221
      tunnel: w234 -> [_ w606 w611 w623 w681 w686 w695 w701 w707 w713 w724 w733 w742 w750 w765 w798 w826 w846 w862 w877 w902 w915 w933 w955 w978 w1014 w1020 w1087 w1092 w1103 w1118 w1131 w1167 w1199]
      tunnel: [w585 w606 w611 w622 w681 w686 w695 w701 w707 w713 w723 w732 w741 w750 w764 w798 w826 w857 w862 w876 w901 w916 w932 w952 w979 w1012 w1042 w1085 w1092 w1103 w1118 w1127 w1168 w1199] -> w229
      tunnel: w233 -> [_ w602 w613 w617 w683 w687 w697 w703 w709 w715 w720 w729 w738 w747 w762 w800 w828 w859 w865 w879 w899 w918 w935 w956 w980 w1015 w1044 w1089 w1096 w1107 w1122 w1133 w1170 w1202]
      tunnel: w223 -> [_ _ w612 w619 _ _ _ _ _ _ _ _ _ _ _ _ _ _ _ _ _ _ _ w953 w963 _ w1043 w1084 _ _ _ w1128 w1166 _]
      tunnel: [_ _ w612 _ _ _ _ _ _ _ _ _ _ _ _ _ _ _ _ _ _ _ _ _ _ _ _ _ _ _ _ _ _ _] -> _
      tunnel: [w573 w604 w610 w620 w679 w689 w692 w700 w706 w712 w721 w730 w739 w748 w763 w801 w829 w858 w861 w878 w900 w917 w934 w954 w981 w1016 w1041 w1086 w1093 w1104 w1113 w1125 w1169 w1200] -> w228
      tunnel: w232 -> [_ w604 w610 w621 w679 w689 w692 w700 w706 w712 w721 w730 w739 w748 w761 w801 w829 w858 w861 w878 w900 w917 w934 w954 w981 w1016 w1041 w1086 w1093 w1104 w1113 w1125 w1169 w1200]
      tunnel: [string[] ["Params.Restore", "ready", "Session.Apply"] string[] ["exit?"] string[] ["exit?"] w618 _ string[] ["Session.New"] _ string[] ["Params.Load:prompt"] string[] ["Params.Save"] string[] ["Params.Save:prompt"] _ _ _ w743 w754 w796 _ _ string[] ["Edit"] _ _ _ _ _ _ _ w1029 _ _ _ _ w1123 _ _] -> w230
      tunnel: [refnum<class "FSM.Graph.lvclass"> refnum ("FSM") w601 w608 w616 w678 w684 w691 w698 w704 w710 w719 w728 w737 w744 w756 w789 w827 w856 w863 w875 w895 w914 w931 w951 w977 w1013 w1033 w1079 w1090 w1101 w1112 w1124 w1165 w1196] -> w219
      tunnel: w217 -> [_ w601 w608 w616 w678 w684 w691 w698 w704 w710 w719 w728 w737 w744 w755 w788 w827 w856 w863 w875 w895 w914 w931 w951 w977 w1013 w1033 w1079 w1090 w1101 w1112 w1124 w1165 w1196]
      event Timeout {
        w568 = FALSE ("Visible")
        w574 = FALSE
        w581 = T32 {"AutoDI"=FALSE, "Max errors"=1, "Headway (%)"=50.0, "DI dt"=2}  # Options
        w584 = FALSE ("Visible")
        w591 = FALSE ("Visible")
        n118 = event-data() -> ()  [unwired: 1 in, 1 out]
        n119 = disable-structure shown="Enabled" {
          disable-tunnel: [w599 string[] ["dafuq", "-rig", "Rig2"] ("App.Args")] -> w567
          frame Enabled {
            n120 = property class="App"() -> ("App.Args"=w599:string[])  [unwired: 2 in, 2 out]
          }
          frame Disabled {
          }
        }
        n121 = call "Tosca-Restore Visual Display Settings.vi"() -> ("Visual Display Settings"=w565:T33)  [unwired: 14 in, 1 out]
        n122 = Unbundle By Name(w565) -> ("Open at start"=w566:bool)
        n123 = control-ref of="Graphs"() -> (w589:refnum<vi>)
        n124 = control-ref of="Status"() -> (w586:refnum<vi>)
        n125 = control-ref of="FSM.Graph"() -> (w554:refnum<vi>)
        n126 = control-ref of="Histogram"() -> (w592:refnum<vi>)
        n127 = control-ref of="Track"() -> (w588:refnum<vi>)
        n128 = control-ref of="Pause"() -> (w569:refnum<vi>)
        n129 = control-ref of="Result"() -> (w593:refnum<vi>)
        n130 = control-ref of="Log"() -> (w587:refnum<vi>)
        n131 = call "Tosca-Parse Application Args.vi"("App.Args"=w567) -> ("config"=w562:string, "rigname"=w553:string, "rignum"=w561:i32, "title"=w563:string)  [unwired: 11 in]
        n132 = control-ref of="Slide"() -> (w594:refnum<vi>)
        n133 = control-ref of="This VI"() -> (w564:refnum<vi>)
        n134 = global write "Tosca-Globals.vi" "Rig"(w553) -> ()
        n135 = case shown="True" w566 {
          tunnel: w565 -> [_ w598]
          frame False {
          }
          frame True {
            n136 = call "Tosca-Open Visual Display.vi"("Visual Display Settings"=w598) -> ("error out"=w597:errorcluster)  [unwired: 14 in]
            n137 = call "Error Handler.vi"("error in (no error)"=w597) -> ()  [unwired: 12 in, 3 out]
          }
        }
        n138 = property class="VI"(reference=w564, "Front Panel.Title"=w563) -> (reference out=w560:refnum<vi>)  [unwired: 1 in, 1 out]
        n139 = call "Tosca-Restore Position.vi"("Config"=w562, "rignum"=w561) -> ("Position"=w558:cluster{"Left":i32, "Top":i32})  [unwired: 12 in, 1 out]
        n140 = global write "Tosca-Globals.vi" "Config"(w562) -> ()
        n141 = call "Tosca-Initialize State.vi"("Config"=w562) -> ("State"=w585:T4)  [unwired: 13 in, 1 out]
        n142 = Bundle("FSM.Graph"=w554, "Slide"=w594, "Result"=w593, "Histogram"=w592, "Graphs"=w589, "Track"=w588, "Log"=w587, "Status"=w586, "Pause"=w569) -> (→"Control Refs":T34)  [unwired: 1 in]
        n143 = call "Set Window Origin.vi"("VI in"=w560) -> ("VI out"=w559:refnum<vi>)  [unwired: 12 in, 2 out]
        n144 = property on="Apply" class="Bool"("Visible"=w584) -> ()  [unwired: 2 in, 2 out]
        n145 = property on="Cancel" class="Bool"("Visible"=w584) -> ()  [unwired: 2 in, 2 out]
        n146 = call "Set Window Position (left, top).vi"("VI in"=w559, "Coords"=w558) -> ()  [unwired: 12 in, 2 out]
        n147 = local write "MATLAB function"(path "" ("MATLAB function")) -> ()
        n148 = call "Error Library.vi"("Priority"=TRUE) -> ()  [unwired: 12 in, 3 out]
        n149 = property on="Pause" class="Bool (strict)"("Visible"=w568, "Blinking"=w568) -> ()  [unwired: 2 in, 2 out]
        n150 = property on="Play" class="Bool"("Visible"=TRUE) -> ()  [unwired: 2 in, 2 out]
        n151 = call "Config File Path.vi"("AppName"=w562) -> ("Default config file name"=w580:path)
        n152 = control-ref of="DIPanel"() -> (w575:refnum<vi>)
        n153 = call "Read Anything.vi"("Type of Anything"=w581, "Path (dialog)"=w580) -> ("Error Out"=w582:errorcluster, "Anything"=w583:variant)  [unwired: 7 in, 1 out]
        n154 = vi-ref "Tosca-DI Thread.vi"() -> (w576:refnum<vi>)
        n155 = property on="Thread Indicators" class="Arr (strict)"("Value"=T1[] [0] ("Thread Indicators"), "Number of Columns"=u32 1) -> ()  [unwired: 2 in, 2 out]
        n156 = Variant To Data(error in=w582, type=w581, Variant=w583) -> (data=w573:T32)  [unwired: 1 out]
        n157 = call "Insert VI in Subpanel.vi"("VI Ref"=w576, "SubPanel"=w575) -> ()  [unwired: 12 in, 2 out]
        n158 = Unbundle By Name(w573) -> ("Max errors"=w572:i32, "Headway (%)"=w571:dbl, "DI dt"=w570:i32)
        n159 = property on="Sched:CS+/CS-" class="Bool"("Visible"=w574) -> ()  [unwired: 2 in, 2 out]
        n160 = property on="Sched:2AFC" class="Bool"("Visible"=w574) -> ()  [unwired: 2 in, 2 out]
        n161 = property on="Histogram" class="XYGraph (strict)"("Visible"=w591) -> ()  [unwired: 2 in, 2 out]
        n162 = property on="Result" class="Str"("Visible"=w591) -> ()  [unwired: 2 in, 2 out]
        n163 = global write "Tosca-Globals.vi" "Max errors"(w572) -> ()
        n164 = global write "Tosca-Globals.vi" "Headway (%)"(w571) -> ()
        n165 = global write "Tosca-Globals.vi" "DI dt"(w570) -> ()
      }
      event Panel Close? {
        n166 = event-data() -> ()  [unwired: 1 in, 1 out]
        n167 = event-data("Discard?"=TRUE) -> ()  [unwired: 1 in, 1 out]
      }
      event "Exit": Value Change {
        n168 = event-data() -> ()  [unwired: 1 in, 1 out]
      }
      event Menu Selection (User) {
        n169 = event-data() -> ("ItemTag"=w624:string)  [unwired: 1 in]
        n170 = case shown="\"mmHelpReset\"" w624 {
          tunnel: [w626 w629 w632 w635 w638 w642 w648 w655 w658 w670 w677] -> w622
          tunnel: w623 -> [w626 w629 w632 w635 w638 w643 w649 w655 w659 w670 w677]
          tunnel: w621 -> [w625 w628 w631 w634 w637 w640 w646 w656 w663 w669 w676]
          tunnel: [w625 w628 w631 w634 w637 w640 w646 w656 w663 w669 w676] -> w620
          tunnel: w619 -> [_ _ _ _ _ _ _ _ w662 _ _]
          tunnel: [_ string[] ["Params.Load:prompt"] string[] ["Params.Save"] string[] ["Params.Save:prompt"] string[] ["exit?"] w639 w645 _ _ _ _] -> w618
          frame "False", Default {
          }
          frame "mmFileLoad" {
          }
          frame "mmFileSave" {
          }
          frame "mmFileSaveAs" {
          }
          frame "mmFileExit" {
          }
          frame "mmEditClearFlowchart" {
            n171 = call "Display Message to User2"() -> ("Yes"=w641:bool)  [unwired: 10 in, 1 out]
            n172 = case shown="True" w641 {
              tunnel: [_ string[] ["Params.ClearFlowchart"]] -> w639
              frame False {
              }
              frame True {
              }
            }
            n173 = Bundle By Name(cluster=w643, "dirty"=w641) -> (w642:T4)
          }
          frame "mmEditClearAll" {
            n174 = call "Display Message to User"() -> ("Yes"=w647:bool)  [unwired: 10 in, 1 out]
            n175 = case shown="True" w647 {
              tunnel: [_ string[] ["Edit", "Params.Clear"]] -> w645
              frame False {
              }
              frame True {
              }
            }
            n176 = Bundle By Name(cluster=w649, "dirty"=w647) -> (w648:T4)
          }
          frame "mmHelpReset" {
            n177 = Two Button Dialog(message="Resetting the hardware will disrupt some other applications, e.g. locomotion tracking.\n\nAre you sure you want to reset the hardware?", 1:"No" ("F button name (\"Cancel\")"), 2:"Yes" ("T button name (\"OK\")")) -> (T button?=w653:bool)
            n178 = case shown="True" w653 {
              frame False {
              }
              frame True {
                n179 = call "PXI-Reset Devices.vi"() -> ()  [unwired: 11 in, 1 out]
              }
            }
          }
          frame "mmHelpMATLAB" {
            n180 = Unbundle By Name(w662) -> ("MATLAB"=w661:refnum<notifier>)
            n181 = Unbundle By Name(w659) -> ("MATLAB"=w660:bool)
            n182 = case shown="False" w660 {
              selector: w660 -> [_ w668]
              tunnel: w661 -> [w667 _]
              tunnel: [w664 w668] -> w657
              frame False {
                n183 = call "Tosca-Start MATLAB Thread.vi"("MATLAB notifier"=w667) -> ("error out"=w666:errorcluster)  [unwired: 14 in]
                n184 = call "Error Handler.vi"("error in (no error)"=w666) -> ("error?"=w665:bool)  [unwired: 12 in, 2 out]
                n185 = Not(x=w665) -> (.not. x?=w664:bool)
              }
              frame True {
              }
            }
            n186 = Bundle By Name(cluster=w659, "MATLAB"=w657) -> (w658:T4)
          }
          frame "mmHelpHelp" {
            n187 = disable-structure shown="RUN_TIME_ENGINE==False" {
              frame condition #0 {
                n188 = call <vilib>:"Application Directory.vi"() -> ("Application Directory"=w673:path)
                n189 = Build Path(base path=w673, name or relative path=path "docs/index.htm") -> (appended path=w671:path)
                n190 = call-poly <vilib>:"Open URL in Default Browser.vi"("path"=w671) -> ()  [unwired: 5 in, 2 out]
              }
              frame condition #1 (active) {
                n191 = Control Online Help(2:path "C:/Users/kehan/OneDrive/Engineering/Help/epl-tosca-help/Tosca Help.chm", 4:enum16{"Contents", "Key", "Close"}."Contents" ("Operation")) -> ()  [unwired: 2 in, 1 out]
              }
            }
          }
          frame "mmHelpAbout" {
            n192 = call "Tosca-Splash Screen.vi"() -> ()  [unwired: 15 in, 1 out]
          }
        }
      }
      event "Session Info": Value Change {
        w680 = TRUE ("Visible")
        n193 = event-data() -> ()  [unwired: 1 in, 1 out]
        n194 = property on="Apply" class="Bool"("Visible"=w680) -> ()  [unwired: 2 in, 2 out]
        n195 = property on="Cancel" class="Bool"("Visible"=w680) -> ()  [unwired: 2 in, 2 out]
      }
      event "Apply": Value Change {
        w688 = FALSE
        n196 = event-data() -> ()  [unwired: 1 in, 1 out]
        n197 = property on="Apply" class="Bool"("Visible"=w688) -> ()  [unwired: 2 in, 2 out]
        n198 = property on="Cancel" class="Bool"("Visible"=w688) -> ()  [unwired: 2 in, 2 out]
      }
      event "Cancel": Value Change {
        w693 = FALSE ("Visible")
        n199 = event-data() -> ()  [unwired: 1 in, 1 out]
        n200 = Unbundle By Name(w695) -> ("Session"=w694:T35)
        n201 = property on="Apply" class="Bool"("Visible"=w693) -> ()  [unwired: 2 in, 2 out]
        n202 = property on="Cancel" class="Bool"("Visible"=w693) -> ()  [unwired: 2 in, 2 out]
        n203 = local write "Session Info"(w694) -> ()
      }
      event "Open": Value Change {
        n204 = event-data() -> ()  [unwired: 1 in, 1 out]
      }
      event "Save": Value Change {
        n205 = event-data() -> ()  [unwired: 1 in, 1 out]
      }
      event "Save as": Value Change {
        n206 = event-data() -> ()  [unwired: 1 in, 1 out]
      }
      event "Description": Value Change {
        n207 = event-data() -> ()  [unwired: 1 in, 1 out]
        n208 = property class="Tosca"(reference=w718, "Accessors:Description"="Description") -> (reference out=w716:refnum<class "Parameters.lvclass">)  [unwired: 1 in, 1 out]
        n209 = Bundle By Name(cluster=w724, "dirty"=TRUE) -> (w723:T4)
      }
      event "MATLAB function": Value Change {
        n210 = event-data() -> ()  [unwired: 1 in, 1 out]
        n211 = property class="Tosca"(reference=w727, "Accessors:MATLAB function"="MATLAB function") -> (reference out=w725:refnum<class "Parameters.lvclass">)  [unwired: 1 in, 1 out]
        n212 = Bundle By Name(cluster=w733, "dirty"=TRUE) -> (w732:T4)
      }
      event "Link to": Value Change {
        n213 = event-data() -> ()  [unwired: 1 in, 1 out]
        n214 = property class="Tosca"(reference=w736, "Accessors:Link to"="Link to") -> (reference out=w735:refnum<class "Parameters.lvclass">)  [unwired: 1 in, 1 out]
        n215 = Bundle By Name(cluster=w742, "dirty"=TRUE) -> (w741:T4)
      }
      event "FSM.Graph": Mouse Down {
        n216 = event-data() -> ("Mods.Double Click"=w752:bool)  [unwired: 1 in]
        n217 = Unbundle By Name(w750) -> ("Measuring"=w749:bool)
        n218 = Not(x=w749) -> (.not. x?=w746:bool)
        n219 = And(x=w746, y=w752) -> (x .and. y?=w745:bool)
        n220 = case shown="True" w745 {
          tunnel: [_ string[] ["Edit"]] -> w743
          frame False {
          }
          frame True {
          }
        }
      }
      event "General Options": Value Change {
        n221 = event-data() -> ()  [unwired: 1 in, 1 out]
        n222 = call "Tosca-Setup General Options.vi"("Options In"=w761) -> ("Options Out"=w759:T32, "Canceled?"=w760:bool)  [unwired: 13 in]
        n223 = Unbundle By Name(w761) -> ("AutoDI"=w758:bool)
        n224 = case shown="False" w760 {
          tunnel: [w782 w787] -> w757
          tunnel: w766 -> [w782 w787]
          tunnel: [w781 w786] -> w764
          tunnel: w765 -> [w771 w786]
          tunnel: [w774 w785] -> w763
          tunnel: w761 -> [_ w785]
          tunnel: w759 -> [w774 _]
          tunnel: w758 -> [w776 _]
          tunnel: [w769 w784] -> w756
          tunnel: w755 -> [w769 w784]
          tunnel: [w767 _] -> w754
          frame False {
            n225 = Unbundle By Name(w771) -> ("Config"=w770:path)
            n226 = Unbundle By Name(w774) -> ("AutoDI"=w778:bool)
            n227 = Unbundle By Name(w774) -> ("Max errors"=w775:i32, "Headway (%)"=w773:dbl, "DI dt"=w772:i32)
            n228 = call "Write Anything.vi"("Section Name (Name of \"Anything\")"="Options" ("Section Name (Name of \"Anything\")"), "Anything"=w774, "Path (dialog)"=w770) -> ()  [unwired: 7 in, 2 out]
            n229 = Not(x=w776) -> (.not. x?=w777:bool)
            n230 = And(x=w778, y=w777) -> (x .and. y?=w768:bool)
            n231 = case shown="True" w768 {
              tunnel: [_ string[] ["DI.Start"]] -> w767
              frame False {
              }
              frame True {
              }
            }
            n232 = global write "Tosca-Globals.vi" "Max errors"(w775) -> ()
            n233 = global write "Tosca-Globals.vi" "Headway (%)"(w773) -> ()
            n234 = global write "Tosca-Globals.vi" "DI dt"(w772) -> ()
            n235 = Bundle By Name(cluster=w771, "dirty"=TRUE) -> (w781:T4)
          }
          frame True {
          }
        }
      }
      event "Devices": Value Change {
        n236 = event-data() -> ()  [unwired: 1 in, 1 out]
        n237 = property class="Tosca"(reference=w794) -> ("Accessors:Imaging.mode"=w792:T18)  [unwired: 1 in, 2 out]
        n238 = Unbundle By Name(w798) -> ("Config"=w797:path)
        n239 = Equal?(x=w792, y=Tosca-Imaging_Mode."Widefield") -> (x = y?=w790:bool)
        n240 = control-ref of="This VI"() -> (w793:refnum<vi>)
        n241 = call "Tosca-Setup Devices.vi"("Configuration file"=w797, "Parent VI"=w793, "frame trigger?"=w790) -> ("Changed"=w799:bool)  [unwired: 12 in]
        n242 = case shown="True" w799 {
          tunnel: [w803 w806] -> w795
          tunnel: w794 -> [w803 w807]
          tunnel: [_ string[] ["DI.AutoStart", "Show.Redisplay"]] -> w796
          tunnel: w788 -> [w802 w805]
          tunnel: [w802 w804] -> w789
          frame False {
          }
          frame True {
            n243 = call "Tosca-Init Params.vi"("Tosca"=w807, "FSM.Graph"=w805) -> ("Tosca Out"=w806:refnum<class "Parameters.lvclass">, "FSM.Graph Out"=w804:refnum<class "FSM.Graph.lvclass">, "error out"=w809:errorcluster)  [unwired: 11 in]
            n244 = call "Error Handler.vi"("error in (no error)"=w809) -> ()  [unwired: 12 in, 3 out]
          }
        }
      }
      event "Calibration": Value Change {
        n245 = event-data() -> ()  [unwired: 1 in, 1 out]
        n246 = Unbundle By Name(w826) -> ("Config"=w822:path)
        n247 = global read "Tosca-Globals.vi" "Rig"() -> (w819:string)
        n248 = call "CM-Endpoint Name To Device.vim"("Path"=w822, "IO Type"="Analog Inputs", "Names in"="Cal Mic") -> ("Path thru"=w821:path, "Devices"=w812:string, "error out"=w820:errorcluster)  [unwired: 9 in, 1 out]
        n249 = Empty String/Path?(string/path=w819) -> (empty?=w823:bool)
        n250 = case shown="False" w823 {
          tunnel: w819 -> [w842 _]
          tunnel: [w841 ""] -> w816
          frame False {
            n251 = Concatenate Strings("." ("string"), w842) -> (w841:string)
          }
          frame True {
          }
        }
        n252 = call "CM-Endpoint Name To Device.vim"("Path"=w821, "IO Type"="Analog Outputs", "Names in"=string[] [], "error in (no error)"=w820) -> ("Names out"=w818:string[], "Devices"=w817:string[], "error out"=w814:errorcluster)  [unwired: 8 in, 1 out]
        n253 = for {
          tunnel: w818 -> [w837] mode=indexing
          tunnel: w817 -> [w839] mode=indexing
          tunnel: w816 -> [w838]
          tunnel: [w835] -> w813 mode=indexing
          n254 = Concatenate Strings(w839, w838) -> (w836:string)
          n255 = Bundle("String"=w837, w836) -> (w835:cluster{"String":string, string})  [unwired: 1 in]
        }
        n256 = case shown="No Error" w814 {
          selector: w814 -> [_ w834]
          tunnel: path "C:/Data/Tosca/Calibration Files" ("base path") -> [w833 _]
          tunnel: w813 -> [w832 _]
          tunnel: w812 -> [w831 _]
          frame No Error {
            n257 = call "Freefield Calibration.vi"("Folder"=w833, "Endpoints"=w832, "Mic device"=w831) -> ()  [unwired: 13 in]
          }
          frame Error {
            n258 = call "Error Handler.vi"("error in (no error)"=w834) -> ()  [unwired: 12 in, 3 out]
          }
        }
      }
      event "Connect": Value Change {
        n259 = event-data() -> ()  [unwired: 1 in, 1 out]
        n260 = property class="Tosca"(reference=w847) -> (reference out=w850:refnum<class "Parameters.lvclass">, "Accessors:Connect"=w851:T25)  [unwired: 1 in, 1 out]
        n261 = Unbundle By Name(w846) -> ("Config"=w845:path)
        n262 = control-ref of="This VI"() -> (w844:refnum<vi>)
        n263 = call "Tosca-Setup Connections.vi"("Connect"=w851, "Parent VI"=w844, "config path"=w845) -> ("Connect out"=w849:T25, "Canceled?"=w852:bool)  [unwired: 11 in]
        n264 = property class="Tosca"(reference=w850, "Accessors:Connect"=w849) -> (reference out=w848:refnum<class "Parameters.lvclass">)  [unwired: 1 in, 1 out]
        n265 = Unbundle By Name(w846) -> ("dirty"=w854:bool)
        n266 = Not(x=w852) -> (.not. x?=w855:bool)
        n267 = Or(x=w854, y=w855) -> (x .or. y?=w853:bool)
        n268 = Bundle By Name(cluster=w846, "dirty"=w853) -> (w857:T4)
      }
      event "Flowchart": Value Change {
        n269 = event-data() -> ()  [unwired: 1 in, 1 out]
      }
      event "Analog Input": Value Change {
        n270 = event-data() -> ()  [unwired: 1 in, 1 out]
        n271 = property class="Tosca"(reference=w870) -> (reference out=w868:refnum<class "Parameters.lvclass">, "Accessors:AI"=w869:T36)  [unwired: 1 in, 1 out]
        n272 = call "Tosca-Setup Analog Input.vi"("AI in"=w869) -> ("AI out"=w867:T36, "Canceled?"=w871:bool)  [unwired: 13 in]
        n273 = case shown="False" w871 {
          tunnel: w867 -> [w880 _]
          frame False {
            n274 = Unbundle By Name(w880) -> ("active"=w881:bool)
            n275 = case shown="True" w881 {
              tunnel: w880 -> [_ w882]
              frame False {
              }
              frame True {
                n276 = vi-ref "Tosca-Analog Input Thread.vi"() -> (w885:refnum<vi>)
                n277 = call "Spawn VI.vi"("VI reference"=w885) -> ("error out"=w883:errorcluster)  [unwired: 9 in, 1 out]
                n278 = call "Tosca-Send AI Command.vi"("action"="Run", "Variant"=w882, "error in (no error)"=w883) -> ()  [unwired: 12 in, 1 out]
              }
            }
          }
          frame True {
          }
        }
        n279 = property class="Tosca"(reference=w868, "Accessors:AI"=w867) -> (reference out=w866:refnum<class "Parameters.lvclass">)  [unwired: 1 in, 1 out]
        n280 = Unbundle By Name(w877) -> ("dirty"=w874:bool)
        n281 = Not(x=w871) -> (.not. x?=w873:bool)
        n282 = Or(x=w874, y=w873) -> (x .or. y?=w872:bool)
        n283 = Bundle By Name(cluster=w877, "dirty"=w872) -> (w876:T4)
      }
      event "Masker": Value Change {
        n284 = event-data() -> ()  [unwired: 1 in, 1 out]
        n285 = property class="Tosca"(reference=w894) -> (reference out=w892:refnum<class "Parameters.lvclass">, "Accessors:Masker"=w893:refnum<class "Channel.lvclass">, "Accessors:Use masker"=w887:bool)  [unwired: 1 in, 1 out]
        n286 = control-ref of="This VI"() -> (w888:refnum<vi>)
        n287 = call "Tosca-Setup Masker.vi"("Masker in"=w893, "Parent VI"=w888, "Use masker in"=w887) -> ("Masker out"=w891:refnum<class "Channel.lvclass">, "Use masker out"=w886:bool, "Canceled?"=w889:bool)  [unwired: 10 in]
        n288 = property class="Tosca"(reference=w892, "Accessors:Masker"=w891, "Accessors:Use masker"=w886) -> (reference out=w890:refnum<class "Parameters.lvclass">)  [unwired: 1 in, 1 out]
        n289 = Unbundle By Name(w902) -> ("dirty"=w897:bool)
        n290 = Not(x=w889) -> (.not. x?=w898:bool)
        n291 = Or(x=w897, y=w898) -> (x .or. y?=w896:bool)
        n292 = Bundle By Name(cluster=w902, "dirty"=w896) -> (w901:T4)
      }
      event "Scripting": Value Change {
        n293 = event-data() -> ()  [unwired: 1 in, 1 out]
        n294 = property class="Tosca"(reference=w909) -> (reference out=w905:refnum<class "Parameters.lvclass">, "Accessors:Pretrial"=w907:T37, "Accessors:DAQ"=w908:T38)  [unwired: 1 in, 1 out]
        n295 = Unbundle By Name(w908) -> ("AO Fs (Hz)"=w906:dbl)
        n296 = call "Tosca-Setup Pretrial Function.vi"("Pretrial in"=w907, "Fs"=w906) -> ("Pretrial out"=w904:T37, "canceled"=w912:bool)  [unwired: 12 in]
        n297 = property class="Tosca"(reference=w905, "Accessors:Pretrial"=w904) -> (reference out=w903:refnum<class "Parameters.lvclass">)  [unwired: 1 in, 1 out]
        n298 = Unbundle By Name(w915) -> ("dirty"=w913:bool)
        n299 = Not(x=w912) -> (.not. x?=w911:bool)
        n300 = Or(x=w913, y=w911) -> (x .or. y?=w910:bool)
        n301 = Bundle By Name(cluster=w915, "dirty"=w910) -> (w916:T4)
      }
      event "Sched:CS+/CS-", "Sched:2AFC", "Sched:Seq": Value Change {
        n302 = event-data() -> ()  [unwired: 1 in, 1 out]
        n303 = call "Tosca-Setup Schedule.vi"("Tosca"=w922) -> ("Tosca out"=w921:refnum<class "Parameters.lvclass">, "Canceled?"=w923:bool)  [unwired: 13 in]
        n304 = property class="Tosca"(reference=w921) -> (reference out=w920:refnum<class "Parameters.lvclass">, "Accessors:Schedule Mode"=w919:T27)  [unwired: 1 in, 1 out]
        n305 = Equal?(x=Tosca-Schedule_Mode."Seq", y=w919) -> (x = y?=w930:bool)
        n306 = Equal?(x=Tosca-Schedule_Mode."Adapt", y=w919) -> (x = y?=w928:bool)
        n307 = Equal?(x=Tosca-Schedule_Mode."CS+/CS-", y=w919) -> (x = y?=w925:bool)
        n308 = property on="Sched:Seq" class="Bool"("Visible"=w930) -> ()  [unwired: 2 in, 2 out]
        n309 = property on="Sched:2AFC" class="Bool"("Visible"=w928) -> ()  [unwired: 2 in, 2 out]
        n310 = property on="Sched:CS+/CS-" class="Bool"("Visible"=w925) -> ()  [unwired: 2 in, 2 out]
        n311 = Not(x=w923) -> (.not. x?=w924:bool)
        n312 = Bundle By Name(cluster=w933, "dirty"=w924) -> (w932:T4)
      }
      event "Imaging": Value Change {
        n313 = event-data() -> ()  [unwired: 1 in, 1 out]
        n314 = property class="Tosca"(reference=w942) -> (reference out=w939:refnum<class "Parameters.lvclass">, "Accessors:Imaging"=w941:T39)  [unwired: 1 in, 1 out]
        n315 = control-ref of="This VI"() -> (w943:refnum<vi>)
        n316 = call "Tosca-Setup Imaging.vi"("Imaging In"=w941, "Parent VI"=w943) -> ("Imaging Out"=w938:T39, "Canceled?"=w950:bool)  [unwired: 12 in]
        n317 = Unbundle By Name(w941) -> ("mode"=w949:T18)
        n318 = Not(x=w950) -> (.not. x?=w947:bool)
        n319 = Unbundle By Name(w938) -> ("mode"=w940:T18)
        n320 = Unbundle By Name(w955) -> ("dirty"=w946:bool)
        n321 = Not Equal?(x=w940, y=w949) -> (x != y?=w948:bool)
        n322 = property class="Tosca"(reference=w939, "Accessors:Imaging"=w938) -> (reference out=w937:refnum<class "Parameters.lvclass">)  [unwired: 1 in, 1 out]
        n323 = Or(x=w946, y=w947) -> (x .or. y?=w945:bool)
        n324 = Unbundle By Name(w953) -> ("2P"=w944:refnum<notifier>)
        n325 = Bundle By Name(cluster=w955, "dirty"=w945) -> (w952:T4)
        n326 = call "Tosca-Update AO Frame Triggers.vi"("Tosca"=w937) -> ("Tosca out"=w936:refnum<class "Parameters.lvclass">)  [unwired: 13 in, 1 out]
        n327 = case shown="True" w948 {
          tunnel: w944 -> [_ w961]
          tunnel: w940 -> [_ w957]
          frame False {
          }
          frame True {
            n328 = Equal?(x=w957, y=Tosca-Imaging_Mode."Two-photon") -> (x = y?=w959:bool)
            n329 = Bundle(w959) -> (w958:cluster{bool})  [unwired: 1 in]
            n330 = Send Notification(notification=w958, notifier=w961) -> ()  [unwired: 1 in, 2 out]
          }
        }
      }
      event "Play", "play": Value Change {
        n331 = event-data() -> ()  [unwired: 1 in, 1 out]
        n332 = call "Tosca-Initialize.vi"("Tosca"=w966, "State"=w978, "IPC"=w963) -> ("Tosca out"=w965:refnum<class "Parameters.lvclass">, "error out"=w973:errorcluster)  [unwired: 11 in]
        n333 = call "Tosca-Flush IPC.vi"("IPC"=w963, "error in (no error)"=w973) -> ("error out"=w971:errorcluster)  [unwired: 13 in]
        n334 = Unbundle By Name(w963) -> ("MATLAB"=w972:refnum<notifier>, "Start"=w976:refnum<notifier>)
        n335 = property class="Tosca"(reference=w965) -> ("Accessors:Input Events"=w968:T9[], "Accessors:Flags"=w967:T40[])  [unwired: 1 in, 2 out]
        n336 = Unbundle By Name(w963) -> ("DI"=w974:refnum<queue>)
        n337 = call "Uses Vision.vi"("Tosca in"=w965) -> ("Uses vision"=w962:bool, "Tosca out"=w964:refnum<class "Parameters.lvclass">)  [unwired: 8 in, 1 out]
        n338 = call "Tosca-Start DI Thread.vi"("DI"=w974, "Input Events"=w968, "Action"=enum16{"Stop", "Preview", "Run"}."Run", "error in (no error)"=w971, "Flags"=w967) -> ("error out"=w969:errorcluster)  [unwired: 10 in]
        n339 = call "Tosca-Start Threads.vi"("Uses vision"=w962, "IPC"=w963, "error in (no error)"=w969) -> ("error out"=w970:errorcluster)  [unwired: 12 in]
        n340 = case shown="No Error" w970 {
          selector: w970 -> [_ w1010]
          tunnel: w976 -> [w995 _]
          tunnel: w978 -> [w990 w1009]
          tunnel: [w994 w1009] -> w979
          tunnel: w972 -> [w991 _]
          tunnel: w964 -> [w983 _]
          frame No Error {
            w985 = FALSE ("Visible")
            n341 = property class="Tosca"(reference=w983) -> ("Accessors:MATLAB function"=w984:path)  [unwired: 1 in, 2 out]
            n342 = Unbundle By Name(w990) -> ("MATLAB"=w988:bool)
            n343 = flat-sequence {
              tunnel: [w1005] -> w996
              tunnel: w986 -> [w1005]
              frame #0 {
                n344 = local read "Session Info"() -> (w1007:T2)
                n345 = property on="Pause" class="Bool (strict)"("Visible"=TRUE, "Blinking"=FALSE) -> ()  [unwired: 2 in, 2 out]
                n346 = Unbundle By Name(w1007) -> ("Run"=w1006:i32)
                n347 = global write "Tosca-Globals.vi" "Nerror"(0 ("Nerror")) -> ()
                n348 = Increment(x=w1006) -> (x+1=→"Run":i32)
              }
            }
            n349 = Empty String/Path?(string/path=w984) -> (empty?=w992:bool)
            n350 = Or(x=w988, y=w992) -> (x .or. y?=w989:bool)
            n351 = case shown="False" w989 {
              tunnel: w991 -> [w1000 _]
              tunnel: w988 -> [_ w1001]
              tunnel: [TRUE ("MATLAB") w1001] -> w987
              tunnel: [w998 _] -> w986
              frame False {
                n352 = call "Tosca-Start MATLAB Thread.vi"("MATLAB notifier"=w1000) -> ("error out"=w998:errorcluster)  [unwired: 14 in]
              }
              frame True {
              }
            }
            n353 = Send Notification(notification=w983, notifier=w995, error in (no error)=w996) -> (error out=w997:errorcluster)  [unwired: 1 out]
            n354 = Bundle By Name(cluster=w990, "Measuring"=TRUE, "MATLAB"=w987, "aborted"=FALSE) -> (w994:T4)
            n355 = property on="Play" class="Bool"(error in=w997, "Visible"=w985) -> ()  [unwired: 1 in, 2 out]
            n356 = property on="Sched:Seq" class="Bool"("Visible"=w985) -> ()  [unwired: 2 in, 2 out]
          }
          frame Error {
            n357 = call "Error Handler.vi"("error in (no error)"=w1010) -> ()  [unwired: 12 in, 3 out]
          }
        }
      }
      event "Stop": Value Change {
        n358 = event-data() -> ()  [unwired: 1 in, 1 out]
        n359 = case shown="True" "Stop" {
          frame False {
          }
          frame True {
            n360 = call "Tosca-Send Abort.vi"() -> ()  [unwired: 16 in]
          }
        }
        n361 = Bundle By Name(cluster=w1014, "aborted"=TRUE) -> (w1012:T4)
      }
      event "finished": Value Change {
        w1035 = FALSE ("Visible")
        n362 = event-data() -> ("NewVal"=w1026:errorcluster)  [unwired: 1 in]
        n363 = Unbundle By Name(w1043) -> ("DI"=w1040:refnum<queue>, "2P"=w1039:refnum<notifier>)
        n364 = Unbundle By Name(w1020) -> ("active threads"=w1023:T5[])
        n365 = property class="Tosca"(reference=w1031) -> ("Accessors:Link to"=w1025:path)  [unwired: 1 in, 2 out]
        n366 = Unbundle By Name(w1020) -> ("Config"=w1032:path)
        n367 = Unbundle By Name(w1020) -> ("aborted"=w1027:bool)
        n368 = call "Error Handler.vi"("error in (no error)"=w1026) -> ("No Error"=w1036:errorcluster)  [unwired: 12 in, 2 out]
        n369 = invoke on="FSM.Graph" class="FSMGraph (strict)" method="Highlight.vi"() -> ()  [unwired: 4 in, 4 out]
        n370 = call "Tosca-Clear Digital Outputs.vi"("Config path"=w1032, "error in (no error)"=w1036) -> ("error out"=w1037:errorcluster)  [unwired: 13 in]
        n371 = call "FileIO-File or Folder Exists.vi"("path"=w1025) -> ("Exists?"=w1030:bool)  [unwired: 7 in, 3 out]
        n372 = Search 1D Array(1D array=w1023, element=Tosca-Thread_Type."ET") -> (index of element=w1021:i32)  [unwired: 1 in]
        n373 = call "Error Handler.vi"("error in (no error)"=w1037) -> ()  [unwired: 12 in, 3 out]
        n374 = Less Than 0?(x=w1021) -> (x < 0?=w1019:bool)
        n375 = property on="Pause" class="Bool (strict)"("Visible"=w1035, "Blinking"=w1035) -> ()  [unwired: 2 in, 2 out]
        n376 = call "Enable or Gray Out.vi"("Boolean"=w1019) -> ("Disabled"=w1024:T31)
        n377 = property on="Sched:Seq" class="Bool"("Visible"=TRUE ("Value (Signaling)")) -> ()  [unwired: 2 in, 2 out]
        n378 = property on="Stop" class="Bool (strict)"("DisabledEnum"=w1024) -> ()  [unwired: 2 in, 2 out]
        n379 = property on="Play" class="Bool"("Visible"=w1019) -> ()  [unwired: 2 in, 2 out]
        n380 = Compound Arithmetic op=AND(w1030, invert w1027, invert w1026) -> (w1028:bool)
        n381 = case shown="True" w1028 {
          tunnel: w1041 -> [w1064 w1071]
          tunnel: w1040 -> [w1063 w1068]
          tunnel: w1039 -> [w1062 _]
          tunnel: w1020 -> [w1046 _]
          tunnel: w1031 -> [w1045 w1070]
          tunnel: [_ string[] ["Link"]] -> w1029
          frame False {
            n382 = Unbundle By Name(w1046) -> ("active threads"=w1056:T5[])
            n383 = Unbundle By Name(w1064) -> ("AutoDI"=w1061:bool)
            n384 = property class="Tosca"(reference=w1045) -> ("Accessors:Imaging.mode"=w1050:T18)  [unwired: 1 in, 2 out]
            n385 = call "Tosca-Init Flags.vi"("Tosca"=w1045) -> ("Tosca Out"=w1048:refnum<class "Parameters.lvclass">)  [unwired: 13 in, 1 out]
            n386 = Select(t=enum16{"Stop", "Preview", "Run"}."Preview" ("Action"), s=w1061, f=enum16{"Stop", "Preview", "Run"}."Stop") -> (s? t:f=w1058:enum16{"Stop", "Preview", "Run"})
            n387 = Search 1D Array(1D array=w1056, element=Tosca-Thread_Type."Imaging") -> (index of element=w1054:i32)  [unwired: 1 in]
            n388 = property class="Tosca"(reference=w1048) -> ("Accessors:Input Events"=w1049:T9[], "Accessors:Flags"=w1047:T40[])  [unwired: 1 in, 2 out]
            n389 = Equal?(x=w1050, y=Tosca-Imaging_Mode."Two-photon") -> (x = y?=w1053:bool)
            n390 = Less Than 0?(x=w1054) -> (x < 0?=w1052:bool)
            n391 = And(x=w1053, y=w1052) -> (x .and. y?=w1051:bool)
            n392 = call "Tosca-Start DI Thread.vi"("DI"=w1063, "Input Events"=w1049, "Action"=w1058, "Flags"=w1047) -> ()  [unwired: 11 in, 1 out]
            n393 = case shown="True" w1051 {
              tunnel: w1062 -> [_ w1065]
              frame False {
              }
              frame True {
                # "Restart 2P frame thread"
                n394 = Bundle(TRUE) -> (w1067:cluster{bool})  [unwired: 1 in]
                n395 = Send Notification(notification=w1067, notifier=w1065) -> ()  [unwired: 1 in, 2 out]
              }
            }
          }
          frame True {
            n396 = Unbundle By Name(w1071) -> ("AutoDI"=w1077:bool)
            n397 = call "Tosca-Init Flags.vi"("Tosca"=w1070) -> ("Tosca Out"=w1069:refnum<class "Parameters.lvclass">)  [unwired: 13 in, 1 out]
            n398 = Select(t=enum16{"Stop", "Preview", "Run"}."Preview" ("Action"), s=w1077, f=enum16{"Stop", "Preview", "Run"}."Stop") -> (s? t:f=w1074:enum16{"Stop", "Preview", "Run"})
            n399 = property class="Tosca"(reference=w1069) -> ("Accessors:Input Events"=w1073:T9[], "Accessors:Flags"=w1072:T40[])  [unwired: 1 in, 2 out]
            n400 = call "Tosca-Start DI Thread.vi"("DI"=w1068, "Input Events"=w1073, "Action"=w1074, "Flags"=w1072) -> ()  [unwired: 11 in, 1 out]
          }
        }
        n401 = Bundle By Name(cluster=w1020, "Measuring"=FALSE) -> (w1042:T4)
      }
      event User Event {
        n402 = event-data() -> ("Running"=w1081:bool)  [unwired: 1 in]
        n403 = Unbundle By Name(w1084) -> ("Events.Threads"=w1083:refnum<user-event>)
        n404 = Bundle("Thread Type"=Tosca-Thread_Type."DI", "Running"=w1081) -> (w1080:cluster{"Thread Type":T5, "Running":bool})  [unwired: 1 in]
        n405 = Generate User Event(user event=w1083, event data cluster=w1080) -> ()  [unwired: 2 in, 2 out]
        n406 = Bundle By Name(cluster=w1087, "DI running"=w1081) -> (w1085:T4)
      }
      event "DI": Value Change {
        n407 = event-data() -> ("NewVal"=w1094:errorcluster)  [unwired: 1 in]
        n408 = Unbundle By Name(w1092) -> ("Measuring"=w1091:bool)
        n409 = case shown="True" w1091 {
          tunnel: w1094 -> [w1097 w1099]
          frame False {
            n410 = disable-structure shown="Disabled" {
              disable-tunnel: w1097 -> [w1098 _]
              frame Disabled {
                n411 = call "Error Handler.vi"("error in (no error)"=w1098) -> ()  [unwired: 12 in, 3 out]
              }
              frame Enabled {
              }
            }
          }
          frame True {
            n412 = case shown="Error" w1099 {
              selector: w1099 -> [_ w1100]
              frame No Error {
              }
              frame Error {
                n413 = call "Error Handler.vi"("error in (no error)"=w1100) -> ()  [unwired: 12 in, 3 out]
                n414 = call "Tosca-Send Abort.vi"() -> ()  [unwired: 16 in]
              }
            }
          }
        }
      }
      event "AI": Value Change {
        n415 = event-data() -> ("NewVal"=w1105:errorcluster)  [unwired: 1 in]
        n416 = Unbundle By Name(w1103) -> ("Measuring"=w1102:bool)
        n417 = case shown="True" w1102 {
          tunnel: w1105 -> [w1108 w1110]
          frame False {
            n418 = disable-structure shown="Disabled" {
              disable-tunnel: w1108 -> [w1109 _]
              frame Disabled {
                n419 = call "Error Handler.vi"("error in (no error)"=w1109) -> ()  [unwired: 12 in, 3 out]
              }
              frame Enabled {
              }
            }
          }
          frame True {
            n420 = case shown="Error" w1110 {
              selector: w1110 -> [_ w1111]
              frame No Error {
              }
              frame Error {
                n421 = call "Error Handler.vi"("error in (no error)"=w1111) -> ()  [unwired: 12 in, 3 out]
                n422 = call "Tosca-Send Abort.vi"() -> ()  [unwired: 16 in]
              }
            }
          }
        }
      }
      event "DI dummy": Shortcut Menu Activation? {
        n423 = event-data() -> ("MenuRef"=w1120:refnum<k9>)  [unwired: 1 in]
        n424 = Unbundle By Name(w1118) -> ("Measuring"=w1116:bool, "DI running"=w1117:bool)
        n425 = Not(x=w1116) -> (.not. x?=w1115:bool)
        n426 = Set Menu Item Info(6:w1117, 7:"diRun" ("item tag"), 9:w1115, 11:w1120) -> ()  [unwired: 3 in, 2 out]
        n427 = event-data("Discard?"=FALSE) -> ()  [unwired: 1 in, 1 out]
      }
      event "DI dummy": Shortcut Menu Selection (User) {
        n428 = event-data() -> ("ItemTag"=w1129:string)  [unwired: 1 in]
        n429 = Unbundle By Name(w1131) -> ("DI running"=w1130:bool)
        n430 = case shown="\"diRun\"" w1129 {
          tunnel: w1130 -> [w1134 w1138]
          tunnel: w1128 -> [_ w1137]
          tunnel: [w1134 FALSE] -> w1126
          tunnel: [_ w1135] -> w1123
          frame "False", Default {
          }
          frame "diRun" {
            n431 = case shown="False" w1138 {
              tunnel: w1137 -> [_ w1140]
              tunnel: [string[] ["DI.Start"] _] -> w1135
              frame False {
              }
              frame True {
                n432 = Unbundle By Name(w1140) -> ("DI"=w1142:refnum<queue>)
                n433 = Enqueue Element(queue=w1142, element=T8 {"Action"=enum."Stop", "Input Events"=[]}) -> ()  [unwired: 2 in, 3 out]
              }
            }
          }
        }
        n434 = Bundle By Name(cluster=w1131, "DI running"=w1126) -> (w1127:T4)
      }
      event User Event {
        n435 = event-data() -> ("ID"=w1147:T5, "Running"=w1145:bool)  [unwired: 1 in]
        n436 = Unbundle By Name(w1166) -> ("MATLAB"=w1154:refnum<notifier>)
        n437 = property class="Tosca"(reference=w1152) -> ("Accessors:MATLAB function"=w1151:path, "Accessors:Connect"=w1150:T25)  [unwired: 1 in, 2 out]
        n438 = Unbundle By Name(w1167) -> ("MATLAB"=w1156:bool)
        n439 = Unbundle By Name(w1167) -> ("active threads"=w1164:T5[])
        n440 = Equal?(x=Tosca-Thread_Type."ET", y=w1147) -> (x = y?=w1144:bool)
        n441 = Empty String/Path?(string/path=w1151) -> (empty?=w1155:bool)
        n442 = Unbundle By Name(w1150) -> ("Synapse"=w1148:bool, "Retrieve"=w1149:bool)
        n443 = Not(x=w1145) -> (.not. x?=w1146:bool)
        n444 = And(x=w1146, y=w1144) -> (x .and. y?=w1143:bool)
        n445 = Search 1D Array(1D array=w1164, element=w1147) -> (index of element=w1162:i32)  [unwired: 1 in]
        n446 = Compound Arithmetic op=AND(invert w1145, w1144, w1156, invert w1155, w1148, w1149) -> (w1153:bool)
        n447 = Greater Or Equal To 0?(x=w1162) -> (x >= 0?=w1163:bool)
        n448 = case shown="False" w1145 {
          tunnel: w1164 -> [w1181 w1191]
          tunnel: w1163 -> [w1182 w1190]
          tunnel: [w1180 w1189] -> w1161
          tunnel: w1147 -> [_ w1188]
          tunnel: w1162 -> [w1179 _]
          frame False {
            n449 = case shown="True" w1182 {
              tunnel: w1181 -> [w1183 w1187]
              tunnel: [w1183 w1186] -> w1180
              tunnel: w1179 -> [_ w1185]
              frame False {
              }
              frame True {
                n450 = Delete From Array(array=w1187, length=1, index=w1185) -> (array with subset deleted=w1186:T5[])  [unwired: 1 out]
              }
            }
          }
          frame True {
            n451 = case shown="False" w1190 {
              tunnel: w1191 -> [w1194 w1195]
              tunnel: [w1192 w1195] -> w1189
              tunnel: w1188 -> [w1193 _]
              frame False {
                n452 = Build Array (concatenate)(w1194, w1193) -> (w1192:T5[])
              }
              frame True {
              }
            }
          }
        }
        n453 = case shown="True" w1153 {
          tunnel: w1154 -> [_ w1176]
          tunnel: w1151 -> [_ w1174]
          frame False {
          }
          frame True {
            n454 = Bundle("Accessors:MATLAB function"=w1174, path "finish") -> (w1175:cluster{"Accessors:MATLAB function":path, path})  [unwired: 1 in]
            n455 = Send Notification(notification=w1175, notifier=w1176) -> ()  [unwired: 1 in, 2 out]
          }
        }
        n456 = Empty Array?(array=w1161) -> (empty?=w1160:bool)
        n457 = Bundle By Name(cluster=w1167, "active threads"=w1161) -> (w1168:T4)
        n458 = case shown="True" w1160 {
          tunnel: w1161 -> [w1177 _]
          tunnel: [w1177 w1178] -> w1158
          frame False {
          }
          frame True {
            w1178 = T5[] [enum."None"] items=["None", "AODO", "Masker", "ET", "Imaging", "Pupil", "AI", "DI", "Camera", "TTL out", "Loco", "Visual"] ("active threads")
          }
        }
        n459 = case shown="True" w1143 {
          frame False {
          }
          frame True {
            n460 = property on="Stop" class="Bool (strict)"("DisabledEnum"=T31."Enabled" ("Disabled")) -> ()  [unwired: 2 in, 2 out]
            n461 = property on="Play" class="Bool"("Visible"=TRUE) -> ()  [unwired: 2 in, 2 out]
          }
        }
        n462 = Array Size(array=w1158) -> (size(s)=w1159:i32)
        n463 = property on="Thread Indicators" class="Arr (strict)"("Value"=w1158, "Number of Columns"=w1159) -> ()  [unwired: 2 in, 2 out]
      }
      event "2P": Value Change {
        n464 = event-data() -> ("NewVal"=w1197:errorcluster)  [unwired: 1 in]
        n465 = Unbundle By Name(w1199) -> ("Measuring"=w1198:bool)
        n466 = case shown="True" w1198 {
          tunnel: w1197 -> [w1203 w1204]
          frame False {
            n467 = call "Error Handler.vi"("error in (no error)"=w1203) -> ()  [unwired: 12 in, 3 out]
          }
          frame True {
            n468 = call "Tosca-Send Error Message.vi"("error in (no error)"=w1204) -> ()  [unwired: 15 in]
          }
        }
      }
    }
    n469 = while {
      shift-right: [w251] -> _
      shift-left: w230 -> [w253]
      shift-right: [w249] -> w220
      shift-left: w221 -> [w248]
      shift-right: [w247] -> w227
      shift-left: w229 -> [w246]
      shift-right: [w245] -> w226
      shift-left: w228 -> [w244]
      tunnel: [w243] -> w225
      tunnel: w223 -> [w242]
      tunnel: w224 -> [w241]
      shift-right: [w237] -> w218
      shift-left: w219 -> [w236]
      stop <- w250 stop-if-true
      n470 = Delete From Array(array=w253) -> (deleted portion=w240:string, array with subset deleted=w252:string[])  [unwired: 2 in]
      n471 = call "Text-Parse String Fields.vi"("String"=w240) -> ("element"=w239:string, "element 2"=w238:string)  [unwired: 9 in, 4 out]
      n472 = case shown="\"exit\"" w239 {
        tunnel: w252 -> [w258 w266 w276 w301 w311 w322 w336 w361 w404 w424 w431 w444 w477 w508 w527 w537 w551]
        tunnel: [w258 w260 w276 w286 w304 w318 w332 w357 w395 w424 w431 w444 w460 w508 w527 w532 w551] -> w251
        tunnel: [w257 w265 w271 w289 w308 w314 w328 w360 w403 w411 w430 w443 w476 w505 w526 w530 w550] -> w249
        tunnel: w248 -> [w257 w265 w271 w292 w308 _ w329 w341 w403 w411 w430 w443 w476 w505 w526 w530 w550]
        tunnel: [w256 w263 w272 w287 w305 w316 w326 w359 w396 w412 w429 w439 w461 w507 w511 w535 w549] -> w247
        tunnel: w246 -> [w256 w263 w272 w288 w306 w320 w334 w356 w396 w413 w429 w439 w462 w507 w511 w535 w549]
        tunnel: [w255 w262 w275 w300 w310 w321 w335 w358 w402 w423 w428 w442 w475 w506 w512 w536 w548] -> w245
        tunnel: w244 -> [w255 w262 w275 w300 w310 w321 w335 w362 w402 w423 w428 w442 w475 w506 w512 w536 w548]
        tunnel: [_ _ _ _ _ _ _ _ _ _ _ _ _ _ TRUE _ _] -> w243
        tunnel: w242 -> [_ _ w270 _ _ _ _ w355 _ _ _ _ _ _ w524 _ _]
        tunnel: w241 -> [_ _ _ _ _ _ _ _ _ _ _ _ _ _ w523 _ _]
        tunnel: w238 -> [_ _ _ _ _ _ _ w363 _ w415 _ w436 _ _ _ _ _]
        tunnel: [w254 w264 w274 w290 w309 refnum<class "FSM.Graph.lvclass"> refnum ("FSM") refnum<class "FSM.Graph.lvclass"> refnum ("FSM") w346 w393 w410 w427 w432 w456 w500 w516 w529 w547] -> w237
        tunnel: w236 -> [w254 w264 w274 w291 w309 _ _ w345 w393 w410 w427 w432 w456 w500 w516 w529 w547]
        frame "", Default {
        }
        frame "DI.AutoStart" {
          n473 = Unbundle By Name(w262) -> ("AutoDI"=w261:bool)
          n474 = case shown="True" w261 {
            tunnel: [_ string[] ["DI.Start"]] -> w259
            frame False {
            }
            frame True {
            }
          }
          n475 = Build Array (concatenate)(w266, w259) -> (w260:string[])
        }
        frame "DI.Start" {
          n476 = Unbundle By Name(w272) -> ("Measuring"=w273:bool)
          n477 = Not(x=w273) -> (.not. x?=w268:bool)
          n478 = Unbundle By Name(w270) -> ("DI"=w269:refnum<queue>)
          n479 = case shown="True" w268 {
            tunnel: w269 -> [_ w283]
            tunnel: w271 -> [_ w280]
            frame False {
            }
            frame True {
              n480 = call "Tosca-Init Flags.vi"("Tosca"=w280) -> ("Tosca Out"=w279:refnum<class "Parameters.lvclass">)  [unwired: 13 in, 1 out]
              n481 = property class="Tosca"(reference=w279) -> ("Accessors:Input Events"=w278:T9[], "Accessors:Flags"=w277:T40[])  [unwired: 1 in, 2 out]
              n482 = call "Tosca-Start DI Thread.vi"("DI"=w283, "Input Events"=w278, "Action"=enum16{"Stop", "Preview", "Run"}."Preview", "Flags"=w277) -> ("error out"=w281:errorcluster)  [unwired: 11 in]
              n483 = call "Error Handler.vi"("error in (no error)"=w281) -> ()  [unwired: 12 in, 3 out]
            }
          }
        }
        frame "Edit" {
          n484 = global read "Tosca-Globals.vi" "Cal folder"() -> (w284:path)
          n485 = Unbundle By Name(w288) -> ("dirty"=w295:bool)
          n486 = control-ref of="This VI"() -> (w293:refnum<vi>)
          n487 = call "Tosca-Editor.vi"("Tosca"=w292, "Parent VI"=w293, "FSM In"=w291, "Cal Folder"=w284) -> ("Tosca out"=w289:refnum<class "Parameters.lvclass">, "FSM out"=w290:refnum<class "FSM.Graph.lvclass">, "canceled"=w294:bool)  [unwired: 9 in]
          n488 = Not(x=w294) -> (.not. x?=w297:bool)
          n489 = Select(t=string[] ["DI.AutoStart", "Show.Redisplay"], s=w297, f=string[] []) -> (s? t:f=w285:string[])
          n490 = Or(x=w297, y=w295) -> (x .or. y?=w296:bool)
          n491 = Bundle By Name(cluster=w288, "dirty"=w296) -> (w287:T4)
          n492 = Build Array (concatenate)(w301, w285) -> (w286:string[])
        }
        frame "Link" {
          n493 = property class="Tosca"(reference=w308) -> ("Accessors:Link to"=w307:path)  [unwired: 1 in, 2 out]
          n494 = Bundle By Name(cluster=w306, "Restore.Params"=w307) -> (w305:T4)
          n495 = for {
            N: 500 -> [_]
            n496 = Wait (ms)(milliseconds to wait=u32 10) -> ()  [unwired: 1 out]
          }
          n497 = Build Array (concatenate)(w311, string[] ["Play", "Params.Load"] ("array")) -> (w304:string[])
        }
        frame "Params.Clear" {
          w315 = path "" ("Parameter file")
          n498 = disable-structure shown="Disabled" {
            disable-tunnel: w320 -> [w324 _]
            frame Disabled {
              n499 = Unbundle By Name(w324) -> ("Config"=w323:path)
              n500 = call "GenCM-List Connected Signals.vi"("Path"=w323) -> ()  [unwired: 10 in, 5 out]
            }
            frame Enabled {
            }
          }
          n501 = local write "Description"("" ("Description")) -> ()
          n502 = Bundle By Name(cluster=w320, "Restore.Params"=w315) -> (w316:T4)
          n503 = local write "Parameter file"(w315) -> ()
          n504 = call "Create.vi"() -> ("Tosca"=w314:refnum<class "Parameters.lvclass">)  [unwired: 15 in]
          n505 = Build Array (concatenate)(w322, "Show.Redisplay" ("String")) -> (w318:string[])
        }
        frame "Params.ClearFlowchart" {
          w325 = path "" ("Parameter file")
          n506 = Bundle By Name(cluster=w334, "Restore.Params"=w325) -> (w326:T4)
          n507 = local write "Parameter file"(w325) -> ()
          n508 = local write "Description"("" ("Description")) -> ()
          n509 = property class="Tosca"(reference=w329, "Accessors:Flowchart"=refnum<class "State.lvclass">[] [] ("Flowchart")) -> (reference out=w328:refnum<class "Parameters.lvclass">)  [unwired: 1 in, 1 out]
          n510 = Build Array (concatenate)(w336, "Show.Redisplay") -> (w332:string[])
        }
        frame "Params.Load" {
          n511 = Unbundle By Name(w356) -> ("Restore.Params"=w354:path)
          n512 = Equal?(x=w363, y="prompt") -> (x = y?=w353:bool)
          n513 = call "Tosca-Read Parameters.vi"("Path in"=w354, "Prompt? (F)"=w353) -> ("Path out"=w350:path, "Tosca"=w339:refnum<class "Parameters.lvclass">, "FSM.Graph"=w344:refnum<class "FSM.Graph.lvclass">, "Loaded?"=w349:bool, "error out"=w348:errorcluster)  [unwired: 9 in]
          n514 = property class="Tosca"(reference=w339) -> ("Accessors:Schedule Mode"=w347:T27, "Accessors:MATLAB function"=w343:path, "Accessors:Link to"=w337:path, "Accessors:Imaging.mode"=w340:T18)  [unwired: 1 in, 2 out]
          n515 = local write "Parameter file"(w350) -> ()
          n516 = call "Error Handler.vi"("error in (no error)"=w348) -> ()  [unwired: 12 in, 3 out]
          n517 = property class="Tosca"(reference=w341) -> ("Accessors:Imaging.mode"=w338:T18)  [unwired: 1 in, 2 out]
          n518 = Bundle By Name(cluster=w356, "Restore.Params"=w350) -> (w351:T4)
          n519 = Not Equal?(x=w340, y=w338) -> (x != y?=w342:bool)
          n520 = case shown="True" w349 {
            tunnel: w341 -> [w374 _]
            tunnel: w351 -> [w373 w392]
            tunnel: [w374 w378] -> w360
            tunnel: [w373 w391] -> w359
            tunnel: w345 -> [w370 _]
            tunnel: w362 -> [w372 w389]
            tunnel: [w372 w389] -> w358
            tunnel: w347 -> [_ w384]
            tunnel: w361 -> [w371 w381]
            tunnel: [w371 w380] -> w357
            tunnel: [w370 w375] -> w346
            tunnel: w339 -> [_ w378]
            tunnel: w344 -> [_ w375]
            tunnel: w343 -> [_ w377]
            tunnel: w337 -> [_ w376]
            frame False {
            }
            frame True {
              n521 = local write "MATLAB function"(w377) -> ()
              n522 = local write "Link to"(w376) -> ()
              n523 = Build Array (concatenate)(w381, string[] ["DI.AutoStart", "Show.Redisplay"]) -> (w380:string[])
              n524 = Equal?(x=Tosca-Schedule_Mode."Seq", y=w384) -> (x = y?=w388:bool)
              n525 = Equal?(x=Tosca-Schedule_Mode."Adapt", y=w384) -> (x = y?=w386:bool)
              n526 = Equal?(x=Tosca-Schedule_Mode."CS+/CS-", y=w384) -> (x = y?=w382:bool)
              n527 = property on="Sched:Seq" class="Bool"("Visible"=w388) -> ()  [unwired: 2 in, 2 out]
              n528 = property on="Sched:2AFC" class="Bool"("Visible"=w386) -> ()  [unwired: 2 in, 2 out]
              n529 = property on="Sched:CS+/CS-" class="Bool"("Visible"=w382) -> ()  [unwired: 2 in, 2 out]
              n530 = Bundle By Name(cluster=w392, "dirty"=FALSE) -> (w391:T4)
            }
          }
          n531 = case shown="True" w342 {
            tunnel: w355 -> [_ w366]
            tunnel: w340 -> [_ w364]
            frame False {
            }
            frame True {
              n532 = Equal?(x=w364, y=Tosca-Imaging_Mode."Two-photon") -> (x = y?=w368:bool)
              n533 = Unbundle By Name(w366) -> ("2P"=w365:refnum<notifier>)
              n534 = Bundle(w368) -> (w367:cluster{bool})  [unwired: 1 in]
              n535 = Send Notification(notification=w367, notifier=w365) -> ()  [unwired: 1 in, 2 out]
            }
          }
        }
        frame "Params.Restore" {
          n536 = Unbundle By Name(w396) -> ("Restore.Params"=w400:path)
          n537 = call <vilib>:"Check if File or Folder Exists.vi"("path"=w400) -> ("file or folder exists?"=w399:bool)  [unwired: 8 in, 2 out]
          n538 = Empty String/Path?(string/path=w400) -> (empty?=w397:bool)
          n539 = Not(x=w397) -> (.not. x?=w398:bool)
          n540 = And(x=w398, y=w399) -> (x .and. y?=w401:bool)
          n541 = case shown="False" w401 {
            tunnel: ["Params.Clear" "Params.Load"] -> w394
            frame False {
            }
            frame True {
            }
          }
          n542 = Build Array (concatenate)(w404, w394) -> (w395:string[])
        }
        frame "Params.Save" {
          n543 = Unbundle By Name(w413) -> ("Restore.Params"=w409:path)
          n544 = Unbundle By Name(w413) -> ("dirty"=w418:bool)
          n545 = Equal?(x=w415, y="prompt") -> (x = y?=w414:bool)
          n546 = Empty String/Path?(string/path=w409) -> (empty?=w407:bool)
          n547 = Or(x=w407, y=w414) -> (x .or. y?=w408:bool)
          n548 = call "Tosca-Write Parameters.vi"("Path in"=w409, "Tosca"=w411, "FSM.Graph"=w410, "Prompt (T)"=w408) -> ("Path out"=w422:path, "Saved?"=w420:bool, "error out"=w421:errorcluster)  [unwired: 9 in]
          n549 = Select(t=FALSE, s=w420, f=w418) -> (s? t:f=w419:bool)
          n550 = local write "Parameter file"(w422) -> ()
          n551 = Bundle By Name(cluster=w413, "dirty"=w419, "Restore.Params"=w422) -> (w412:T4)
          n552 = call "Error Handler.vi"("error in (no error)"=w421) -> ()  [unwired: 12 in, 3 out]
          n553 = case shown="True" w420 {
            frame False {
            }
            frame True {
              n554 = One Button Dialog(message="Parameter file saved.") -> ()  [unwired: 1 in, 1 out]
            }
          }
        }
        frame "Play" {
          n555 = property on="play" class="Bool (strict)"("Val(Sgnl)"=TRUE ("Value (Signaling)")) -> ()  [unwired: 2 in, 2 out]
        }
        frame "Session.Apply" {
          n556 = Unbundle By Name(w439) -> ("Session"=w438:T35, "Session.Path"=w437:path)
          n557 = call "FileIO-File or Folder Exists.vi"("path"=w437) -> ("Directory?"=w434:bool, "dup path"=w435:path)  [unwired: 7 in, 2 out]
          n558 = case shown="False" w434 {
            tunnel: w435 -> [w455 _]
            tunnel: [w454 _] -> w433
            frame False {
              n559 = Create Folder(path (use dialog)=w455) -> (error out=w454:errorcluster)  [unwired: 2 in, 2 out]
            }
            frame True {
            }
          }
          n560 = case shown="No Error" w433 {
            selector: w433 -> [w445 _]
            tunnel: [w452 w453] -> w440
            tunnel: w438 -> [w451 w453]
            tunnel: w436 -> [w450 _]
            frame No Error {
              n561 = call "Tosca-Read Session Info.vi"("Session Info"=w451, "Session Data"=w450, "error in (no error)"=w445) -> ("Session Info out"=w452:T19, "error out"=w448:errorcluster)  [unwired: 11 in]
              n562 = local write "Notes"("" ("Notes")) -> ()
              n563 = call "Filter Error.vi"("error in (no error)"=w448, "code to ignore"=7) -> ("error out"=w446:errorcluster)  [unwired: 9 in]
              n564 = call <vilib>:"Simple Error Handler.vi"("error in (no error)"=w446) -> ()  [unwired: 4 in, 5 out]
            }
            frame Error {
            }
          }
          n565 = local write "Session Info"(w440) -> ()
          n566 = Unbundle By Name(w440) -> ("Run"=w441:i32)
          n567 = local write "Run"(w441) -> ()
        }
        frame "Session.New" {
          n568 = local read "Session Info"() -> (w457:T2)
          n569 = Unbundle By Name(w457) -> ("Subject ID"=w473:string, "Session"=w474:i32)
          n570 = List Folder(path=path "C:/Data/Tosca", pattern="ToscaMetadata.*") -> (path out=w469:path, filenames=w470:string[])  [unwired: 2 in, 2 out]
          n571 = Empty Array?(array=w470) -> (empty?=w465:bool)
          n572 = Format Into String(format string="C:\\\\Data\\\\Tosca\\\\Data\\\\%s\\\\Session %d", w473, w474) -> (resulting string=w472:string)  [unwired: 2 in, 1 out]
          n573 = case shown="False" w465 {
            tunnel: w469 -> [w497 _]
            tunnel: w470 -> [w499 _]
            tunnel: [w496 _] -> w466
            frame False {
              n574 = Index Array(array=w499) -> (element=w498:string)  [unwired: 1 in]
              n575 = Build Path(base path=w497, name or relative path=w498) -> (appended path=w496:path)
            }
            frame True {
            }
          }
          n576 = String To Path(string=w472) -> (path=w463:path)
          n577 = case shown="False" w465 {
            tunnel: [w492 _] -> w458
            tunnel: w457 -> [w495 _]
            tunnel: [w494 _] -> w464
            tunnel: w466 -> [w493 _]
            frame False {
              n578 = call "Tosca-Setup Session Metadata.vi"("Session Info"=w495, "Path"=w493) -> ("Metadata"=w492:string, "Canceled?"=w494:bool)  [unwired: 12 in]
            }
            frame True {
            }
          }
          n579 = case shown="True" w464 {
            tunnel: w463 -> [w486 _]
            tunnel: w462 -> [w485 w491]
            tunnel: [w483 w491] -> w461
            tunnel: [w479 _] -> w459
            tunnel: w458 -> [w481 _]
            tunnel: w457 -> [w478 w490]
            frame False {
              n580 = Bundle By Name(cluster=w478, "Path"=w486) -> (w484:T2)
              n581 = Format Into String(format string="Session.Apply:%s" ("String"), w481) -> (resulting string=w480:string)  [unwired: 2 in, 1 out]
              n582 = Bundle By Name(cluster=w485, "Session"=w484) -> (w483:T4)
              n583 = Build Array(w480) -> (w479:string[])
            }
            frame True {
              n584 = Unbundle By Name(w491) -> ("Session.ID"=w488:string, "Session.Num"=w489:i32)
              n585 = Bundle By Name(cluster=w490, "Subject ID"=w488, "Session"=w489) -> (w487:T2)
              n586 = local write "Session Info"(w487) -> ()
            }
          }
          n587 = Build Array (concatenate)(w477, w459) -> (w460:string[])
        }
        frame "Show.Redisplay" {
          n588 = property class="Tosca"(reference=w505) -> ("Accessors:Schedule Mode"=w503:T27)  [unwired: 1 in, 2 out]
          n589 = local write "Description"("" ("Description")) -> ()
          n590 = Equal?(x=w503, y=Tosca-Schedule_Mode."CS+/CS-") -> (x = y?=w501:bool)
          n591 = property on="FSM.Graph" class="FSMGraph (strict)"("CS+CS-"=w501, "Val(Sgnl)"=w500) -> ()  [unwired: 2 in, 2 out]
        }
        frame "exit" {
          n592 = call "Tosca-Release IPC.vi"("IPC"=w524) -> ()  [unwired: 14 in, 1 out]
          n593 = Unregister For Events(event registration refnum=w523) -> ()  [unwired: 1 in, 1 out]
          n594 = control-ref of="This VI"() -> (w515:refnum<vi>)
          n595 = call "Tosca-Save State.vi"("State"=w511) -> ()  [unwired: 14 in, 1 out]
          n596 = Unbundle By Name(w511) -> ("Config"=w510:path)
          n597 = call "Get Window Position (left, top).vi"("VI in"=w515) -> ("left, top"=w514:cluster{"Left":i16, "Top":i16})  [unwired: 12 in, 2 out]
          n598 = call "Tosca-Restore Visual Display Settings.vi"() -> ("Visual Display Settings"=w520:T33)  [unwired: 14 in, 1 out]
          n599 = Unbundle By Name(w520) -> ("IP Address"=w517:string, "Port"=w518:i32)
          n600 = call "Write Anything.vi"("Section Name (Name of \"Anything\")"="Position" ("Section Name (Name of \"Type of Anything\")"), "Anything"=w514, "Path (dialog)"=w510) -> ()  [unwired: 7 in, 2 out]
          n601 = call "TCP-Send Command.vi"("PXI Address"=w517, "Port"=w518, "Command"="Quit", "timeout (ms)"=100, "byte order"=T30."big-endian, network order") -> ("error out"=w521:errorcluster)  [unwired: 10 in]
          n602 = call <vilib>:"Clear Errors.vi"("error in (no error)"=w521) -> ()  [unwired: 5 in, 2 out]
        }
        frame "exit?" {
          n603 = Unbundle By Name(w535) -> ("Restore.Params"=w528:path, "dirty"=w533:bool, "Measuring"=w534:bool)
          n604 = case shown="False" w534 {
            tunnel: w533 -> [w545 _]
            tunnel: [w541 _] -> w531
            tunnel: w530 -> [w540 _]
            tunnel: w529 -> [w539 _]
            tunnel: w528 -> [w538 _]
            frame False {
              n605 = call "Tosca-Dirty File Check.vi"("Path in"=w538, "Action"="exiting", "Tosca"=w540, "FSM.Graph"=w539, "Is Dirty?"=w545) -> ("Continue?"=w544:bool)  [unwired: 8 in, 2 out]
              n606 = Select(t=string[] ["exit"], s=w544, f=string[] []) -> (s? t:f=w541:string[])
            }
            frame True {
            }
          }
          n607 = Build Array (concatenate)(w537, w531) -> (w532:string[])
        }
        frame "ready" {
          n608 = call "RunExe-Send Target Ready.vi"() -> ()  [unwired: 15 in, 1 out]
        }
      }
      n609 = Empty Array?(array=w251) -> (empty?=w250:bool)
    }
  }
  n610 = call "Tosca-Trace-Logging Thread.vi"("IPC"=w1) -> ()  [unwired: 15 in]
  n611 = disable-structure shown="RUN_TIME_ENGINE==True" {
    disable-tunnel: w18 -> [w1205 _]
    frame condition #0 {
      n612 = Quit LabVIEW(quit? (T)=w1205) -> ()
    }
    frame condition #1 (active) {
    }
  }
